vi "TCP IP Command Tester.vi"() -> ()   [LabVIEW 2015]
uses:
  Controls/Control_Fornax Set Monopolar Command - Coag Mode Enum.ctl
  Controls/Control_Fornax Set Monopolar Command - Serial Number String.ctl
  Controls/Control_Fornax Set Monopolar Command - Energy Channel ID Enum.ctl
  Controls/Control_Fornax Set Monopolar Command - Cut Mode Enum.ctl
  Controls/Control_Fornax Set Monopolar Command - Cut Power Command Enum.ctl
  Controls/Control_Fornax Set Monopolar Command - Coag Power Command Enum.ctl
  Controls/Control_Fornax Source ID.ctl
  Controls/Control_Fornax Switch ID.ctl
  Controls/Control_Fornax Energy Channel ID.ctl
  Controls/Control_Fornax Switch State.ctl
  Controls/Control_Fornax Energy Mode.ctl
  Controls/Control_Fornax Parameter Value.ctl
  Controls/Control_Fornax Parameter Type.ctl
  Controls/Control_Fornax Instrument Type.ctl
  Controls/Control_Fornax Mono1 Cut Increase Power.ctl
  Controls/Control_Fornax Mono1 Cut Decrease Power.ctl
  Controls/Control_Fornax Mono1 Coag Increase Power.ctl
  Controls/Control_Fornax Mono1 Coag Decrease Power.ctl
  Controls/Control_Fornax Mono1 Cut Enum.ctl
  Controls/Control_Fornax Mono1 Coag Enum.ctl
  Controls/Control_Fornax Mono1 Cut Activate Port Bool.ctl
  Controls/Control_Fornax Mono1 Coag Activate Port Bool.ctl
  Controls/Control_Fornax Mono2 Cut Activate Port Bool.ctl
  Controls/Control_Fornax Mono2 Coag Activate Port Bool.ctl
  Controls/Control_Fornax Mono2 Cut Decrease Power.ctl
  Controls/Control_Fornax Mono2 Cut Increase Power.ctl
  Controls/Control_Fornax Mono2 Cut Enum.ctl
  Controls/Control_Fornax Mono2 Coag Decrease Power.ctl
  Controls/Control_Fornax Mono2 Coag Increase Power.ctl
  Controls/Control_Fornax Mono2 Coag Enum.ctl
  Controls/Control_Fornax Bipolar Increase Power.ctl
  Controls/Control_Fornax Bipolar Decrease Power.ctl
  Controls/Control_Fornax Bipolar Enum.ctl
  Controls/Control_Fornax Bipolar Activate Port Bool.ctl
  Controls/Control_Fornax Ligasure Activate Port Bool.ctl
  Controls/QMH Fundamentals - Message Cluster.ctl
  Controls/Control_Fornax Generator.ctl
panel:
  in  "Stop":bool
  in  "Tab Control":T1(tab)
  in  "error in (no error)":errorcluster
  out "output cluster":T2
  out "Array":T3(array[cluster])
  in  "Fornax Executable Path":path=path "C:/Program Files (x86)/Medtronic/Fornax/x86/Fornax.exe"
  in  "Action 1":bool
  in  "ExternalCommCommand":T4(ring)=enum."EXTERNAL_COMM_COMMAND_PAIR_INTEGRATION_TESTOR"
  out "Display Message":string="Wait while TCP Connection established"
  in  "Set Monopolar Command":bool
  in  "CoagMode":T5
  in  "Serial Number":T6="T5G00443DX"
  in  "EnergyChannelID":T7
  in  "CutMode":T8
  in  "CutPowerCommand":T9
  in  "CoagPowerCommand":T10
  out "Display Message page 2":string="Wait while TCP Connection established"
  in  "String Command":string
  in  "Send String Command":bool
  out "String":string
  in  "Numeric (0-8)":i32
  in  "Send String Array Command":bool
  out "status":bool
  out "status 2":bool
  in  "Slider Status Command":bool
  in  "Switch Status Command":bool
  in  "System Config":bool
  in  "External Command":bool
  in  "External Command":T4(ring)
  in  "System Config":T11(ring)
  in  "Source ID":T12
  in  "Switch ID":T13
  in  "Switch State":T14
  in  "Energy Channel ID":T15
  in  "Energy Channel ID 2":T15
  in  "Slider Position":i32
  in  "Energy Parameter Command":bool
  in  "On/Off":bool
  in  "Mode":enum16{"Cut", "Coag", "Bipolar", "Ligasure"}(ring)
  in  "Port":enum16{"Mono1", "Mono2", "Bipolar", "Ligasure"}(ring)
  in  "Energy Mode":T16
  in  "Instrument Type":T17
  in  "Parameter Type":T18
  in  "Parameter Value":T19
  in  "Energy Channel ID 3":T15
  in  "Ligasure Activate":T20
  in  "Bipolar Activate":T21
  in  "Bipolar Enum":T22
  in  "Bipolar minus":T23
  in  "Bipolar plus":T24
  in  "Mono2 Coag Enum":T25=enum."Spray"
  in  "Mono2 Coag plus":T26
  in  "Mono2 Coag minus":T27
  in  "Mono2 Cut Enum":T28
  in  "Mono2 Cut plus":T29
  in  "Mono2 Cut minus":T30
  in  "Mono2 Coag Activate":T31
  in  "Mono2 Cut Activate":T32
  in  "Mono1 Coag Activate":T33
  in  "Mono1 Cut Activate":T34
  in  "Mono1 Coag Enum":T35=enum."Spray"
  in  "Mono1 Cut Enum":T36
  in  "Mono1 Coag minus":T37
  in  "Mono1 Coag plus":T38
  in  "Mono1 Cut minus":T39
  in  "Mono1 Cut plus":T40
  # "Mono1"
  # "Mono2"
  # "Bipolar"
  # "Ligasure"
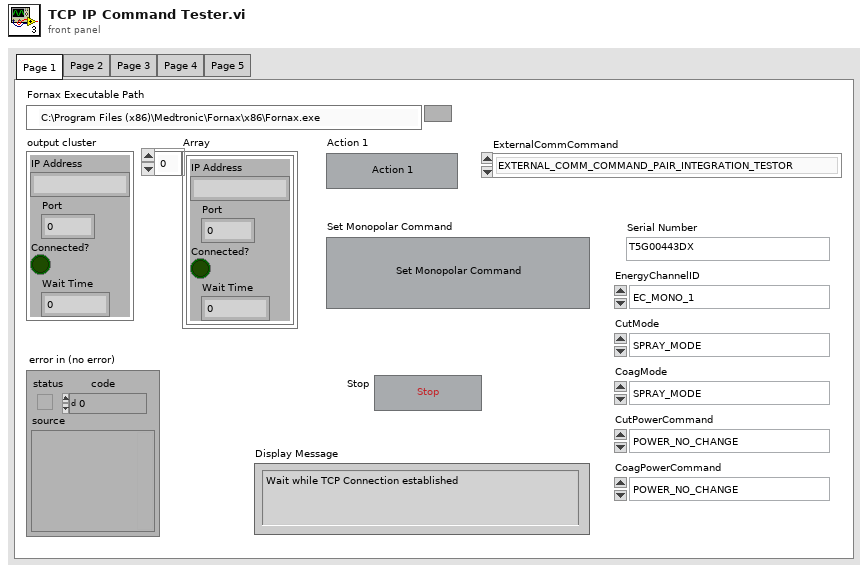
[diagram p1: front panel]
types:
  T1 = enum32{"Page 1", "Page 2", "Page 3", "Page 4", "Page 5"}
  T2 = cluster{"IP Address":string, "Port":u16, "Connected?":bool, "Wait Time":dbl}
  T3 = cluster{"IP Address":string, "Port":u16, "Connected?":bool, "Wait Time":dbl}[]
  T4 = enum16{"EXTERNAL_COMM_COMMAND_INVALID", "EXTERNAL_COMM_COMMAND_PAIR_VLEX", "EXTERNAL_COMM_COMMAND_PAIR_FORNAX", "EXTERNAL_COMM_COMMAND_PAIR_INTEGRATION_TESTOR", "EXTERNAL_COMM_COMMAND_ENABLE_DFA", "EXTERNAL_COMM_COMMAND_ENABLE_DFT", "EXTERNAL_COMM_COMMAND_ENABLE_VIPER", "EXTERNAL_COMM_COMMAND_AUTO_ETHERNET_ON", "EXTERNAL_COMM_COMMAND_AUTO_ETHERNET_OFF", "EXTERNAL_COMM_COMMAND_STREAM_RFDATA_ON", "EXTERNAL_COMM_COMMAND_STREAM_RFDATA_OFF", "EXTERNAL_COMM_COMMAND_STREAM_ISOFIRM_ON", "EXTERNAL_COMM_COMMAND_STREAM_ISOFIRM_OFF", "EXTERNAL_COMM_COMMAND_STREAM_RFID_ON", "EXTERNAL_COMM_COMMAND_STREAM_RFID_OFF", "EXTERNAL_COMM_COMMAND_AUTO_ETHERNET_ONCE"}
  T5 = typedef "Control_Fornax Set Monopolar Command - Coag Mode Enum.ctl" = enum16{"SPRAY_MODE", "CUT_MODE", "BLEND_MODE", "FULGERATE_MODE", "BEPOLAR_MODE", "VESSEL_SEALING_MODE", "VALLEYLAB_MODE", "BIPOLAR_RESECTION_CUT_MODE", "BIPOLAR_RESECTION_COAG_MODE", "AUTOBIPOLAR_MODE", "VIPER_HLA", "SOFT_COAG_MODE", "NUM_ENERGY_MODES"}
  T6 = typedef "Control_Fornax Set Monopolar Command - Serial Number String.ctl" = string
  T7 = typedef "Control_Fornax Set Monopolar Command - Energy Channel ID Enum.ctl" = enum16{"EC_MONO_1", "EC_BIPOLAR", "EC_MONO_2", "EC_ADVANCED", "NUM_ENERGY_CHANNELS", "EC_NOT_USED"}
  T8 = typedef "Control_Fornax Set Monopolar Command - Cut Mode Enum.ctl" = enum16{"SPRAY_MODE", "CUT_MODE", "BLEND_MODE", "FULGERATE_MODE", "BIPOLAR_MODE", "VESSEL_SEALING_MODE", "VALLEYLAB_MODE", "BIPOLAR_RESECTION_CUT_MODE", "BIPOLAR_RESECTION_COAG_MODE", "AUTOBIPOLAR_MODE", "VIPER_HLA", "SOFT_COAG_MODE", "NUM_ENERGY_MODES"}
  T9 = typedef "Control_Fornax Set Monopolar Command - Cut Power Command Enum.ctl" = enum16{"POWER_NO_CHANGE", "POWER_INCREASE", "POWER_DECREASE", "POWER_INCREASE_REPEAT", "POWER_DECREASE_REPEAT"}
  T10 = typedef "Control_Fornax Set Monopolar Command - Coag Power Command Enum.ctl" = enum16{"POWER_NO_CHANGE", "POWER_INCREASE", "POWER_DECREASE", "POWER_INCREASE_REPEAT", "POWER_DECREASE_REPEAT"}
  T11 = enum16{"SYSTEM_CONFIG_CMD_NONE", "SYSTEM_CONFIG_CMD_READ_CONFIG", "SYSTEM_CONFIG_CMD_WRITE_CONFIG", "SYSTEM_CONFIG_CMD_SW_UPDATE_ENTER", "SYSTEM_CONFIG_CMD_SW_UPDATE_START", "SYSTEM_CONFIG_CMD_SW_UPDATE_EXIT", "SYSTEM_CONFIG_CMD_UPDATE_ONE_BOARD_CHASSIS_INFO", "SYSTEM_CONFIG_CMD_UPDATE_ALL_BOARDS_CHASSIS_INFO", "SYSTEM_CONFIG_CMD_READ_ONE_BOARD_INFO", "SYSTEM_CONFIG_CMD_READ_ALL_BOARDS_INFO", "SYSTEM_CONFIG_CMD_REGISTER_BOARD", "SYSTEM_CONFIG_CMD_APPROVE_CURRENT_CONFIG", "SYSTEM_CONFIG_CMD_ROTATE_EVENT_LOGS", "SYSTEM_CONFIG_CMD_SYSTEM_RESTART", "SYSTEM_CONFIG_CMD_ROTATE_USAGE_LOGS", "SYSTEM_CONFIG_CMD_ENTER_SERVICE", "SYSTEM_CONFIG_CMD_EXIT_SERVICE", "SYSTEM_CONFIG_CMD_SW_UPDATE_CONFIRM", "SYSTEM_CONFIG_CMD_ROTATE_ALL_LOGS"}
  T12 = typedef "Control_Fornax Source ID.ctl" = enum16{"SWITCH_SOURCE_UNKNOWN  ", "SWITCH_SOURCE_HANDSWITCH  ", "SWITCH_SOURCE_FOOTSWITCH  ", "SWITCH_SOURCE_AUTO_BIPOLAR  ", "SWITCH_SOURCE_CARDIOBLATE  ", "SWITCH_SOURCE_SCREEN  ", "NUM_SWITCH_SOURCES  "}
  T13 = typedef "Control_Fornax Switch ID.ctl" = enum16{"SWITCH_ID_NONE  ", "SWITCH_ID_CUT  ", "SWITCH_ID_VMODE  ", "SWITCH_ID_COAG  ", "SWITCH_ID_LIGASURE  ", "SWITCH_ID_BIPOLAR  ", "SWITCH_ID_STAPLER_CLOSE  ", "SWITCH_ID_STAPLER_OPEN  ", "SWITCH_ID_CARDIOBLATE_BIPOLAR  ", "SWITCH_ID_CARDIOBLATE_BIPOLAR_TOUCHSCREEN  ", "SWITCH_ID_CARDIOBLATE_MONOPOLAR  ", "SWITCH_ID_CARDIOBLATE_MONOPOLAR_TOUCHSCREEN  ", "SWITCH_ID_ULTRASONIC_BTN1  ", "SWITCH_ID_ULTRASONIC_BTN2  ", "SWITCH_ID_MAX  "}
  T14 = typedef "Control_Fornax Switch State.ctl" = enum16{"SWITCH_STATE_NULL  ", "SWITCH_STATE_PRESSED  ", "SWITCH_STATE_RELEASED  ", "NUM_SWITCH_STATES  "}
  T15 = typedef "Control_Fornax Energy Channel ID.ctl" = enum16{"EC_MONO_1  ", "EC_BIPOLAR  ", "EC_MONO_2  ", "EC_ADVANCED  ", "EC_ADVANCED_ECUT  ", "EC_ADVANCED_DCUT  ", "EC_SHARED_COAG  ", "EC_INTERNAL_BIP_CAL  "}
  T16 = typedef "Control_Fornax Energy Mode.ctl" = enum16{"SPRAY_MODE", "CUT_MODE", "BLEND_MODE", "FULGERATE_MODE", "BIPOLAR_MODE", "VESSEL_SEALING_MODE", "VALLEYLAB_MODE", "BIPOLAR_RESECTION_CUT_MODE", "BIPOLAR_RESECTION_COAG_MODE", "AUTOBIPOLAR_MODE", "VIPER_HLA", "SOFT_COAG_MODE", "ECUT_MODE", "SHARED_SPRAY_MODE", "SHARED_FULGERATE_MODE", "CARDIO_MONO_MODE", "CARDIO_BIPOLAR_MODE", "BIPOLAR_LOW_MODE", "BIPOLAR_MACRO_MODE", "BIPOLAR_STANDARD_MODE", "BIPOLAR_MEDIUM_MODE", "VL_ENDOSCOPY_MODE", "NUM_ENERGY_MODES"}
  T17 = typedef "Control_Fornax Instrument Type.ctl" = enum16{"INSTRUMENT_TYPE_UNKNOWN", "INSTRUMENT_TYPE_MONOPOLAR", "INSTRUMENT_TYPE_BIPOLAR", "INSTRUMENT_TYPE_TRIVERSE", "INSTRUMENT_TYPE_LIGASURE", "INSTRUMENT_TYPE_ADVANCE_II", "INSTRUMENT_TYPE_BIPOLAR_RESECTION", "INSTRUMENT_TYPE_HOOK", "INSTRUMENT_TYPE_BIZACT", "INSTRUMENT_TYPE_CARDIOBLATE_BIP", "INSTRUMENT_TYPE_CARDIOBLATE_BIP_GEMINI_S", "INSTRUMENT_TYPE_CARDIOBLATE_MONO", "INSTRUMENT_TYPE_ULTRASONIC", "INSTRUMENT_TYPE_MONOPOLAR_GI ", "INSTRUMENT_TYPE_GOLDILOCKS "}
  T18 = typedef "Control_Fornax Parameter Type.ctl" = enum16{"POWER_PARAMETER", "CUT_MODALITY_POWER_PARAMETER", "COAG_MODALITY_POWER_PARAMETER", "VL_MODALITY_POWER_PARAMETER", "BY_MODE_POWER_PARAMETER", "VL_ENDO_CUT_MODALITY_POWER_PARAMETER", "VL_ENDO_COAG_MODALITY_POWER_PARAMETER", "VL_ENDO_COAG_ON_CUT_MODALITY_POWER_PARAMETER", "MODE_PARAMETER   (for changing Bipolar mode)", "CUT_MODALITY_MODE_PARAMETER  (for changing monopolar cut mode)", "COAG_MODALITY_MODE_PARAMETER (for changing monopolar coag mode)", "VL_ENDO_COAG_MODALITY_MODE_PARAMETER", "VL_ENDO_CUT_INTERVAL_PARAMETER", "VL_ENDO_CUT_DURATION_PARAMETER", "POWER_BAR_PARAMETER", "MAX_ACTIVATION_MSEC_TIME_PARAMETER", "AUTOBIPOLAR_DELAY_MSEC_TIME", "VL_ENDO_COAG_QUICK_ACCESS_PARAMETER"}
  T19 = typedef "Control_Fornax Parameter Value.ctl" = i32
  T20 = typedef "Control_Fornax Ligasure Activate Port Bool.ctl" = bool
  T21 = typedef "Control_Fornax Bipolar Activate Port Bool.ctl" = bool
  T22 = typedef "Control_Fornax Bipolar Enum.ctl" = enum16{"Standard", "Macro", "Precision"}
  T23 = typedef "Control_Fornax Bipolar Decrease Power.ctl" = bool
  T24 = typedef "Control_Fornax Bipolar Increase Power.ctl" = bool
  T25 = typedef "Control_Fornax Mono2 Coag Enum.ctl" = enum16{"Fulgerate", "Spray"}
  T26 = typedef "Control_Fornax Mono2 Coag Increase Power.ctl" = bool
  T27 = typedef "Control_Fornax Mono2 Coag Decrease Power.ctl" = bool
  T28 = typedef "Control_Fornax Mono2 Cut Enum.ctl" = enum16{"Pure", "Blend"}
  T29 = typedef "Control_Fornax Mono2 Cut Increase Power.ctl" = bool
  T30 = typedef "Control_Fornax Mono2 Cut Decrease Power.ctl" = bool
  T31 = typedef "Control_Fornax Mono2 Coag Activate Port Bool.ctl" = bool
  T32 = typedef "Control_Fornax Mono2 Cut Activate Port Bool.ctl" = bool
  T33 = typedef "Control_Fornax Mono1 Coag Activate Port Bool.ctl" = bool
  T34 = typedef "Control_Fornax Mono1 Cut Activate Port Bool.ctl" = bool
  T35 = typedef "Control_Fornax Mono1 Coag Enum.ctl" = enum16{"Fulgerate", "Spray"}
  T36 = typedef "Control_Fornax Mono1 Cut Enum.ctl" = enum16{"Pure", "Blend"}
  T37 = typedef "Control_Fornax Mono1 Coag Decrease Power.ctl" = bool
  T38 = typedef "Control_Fornax Mono1 Coag Increase Power.ctl" = bool
  T39 = typedef "Control_Fornax Mono1 Cut Decrease Power.ctl" = bool
  T40 = typedef "Control_Fornax Mono1 Cut Increase Power.ctl" = bool
  T41 = typedef "QMH Fundamentals - Message Cluster.ctl" = cluster{"Message":string, "Message Data":variant}
  T42 = cluster{"Port":enum16{"Mono1", "Mono2", "Bipolar", "Ligasure"}, "Mode":enum16{"Cut", "Coag", "Bipolar", "Ligasure"}, "On/Off":bool}
  T43 = typedef "Control_Fornax Generator.ctl" = string
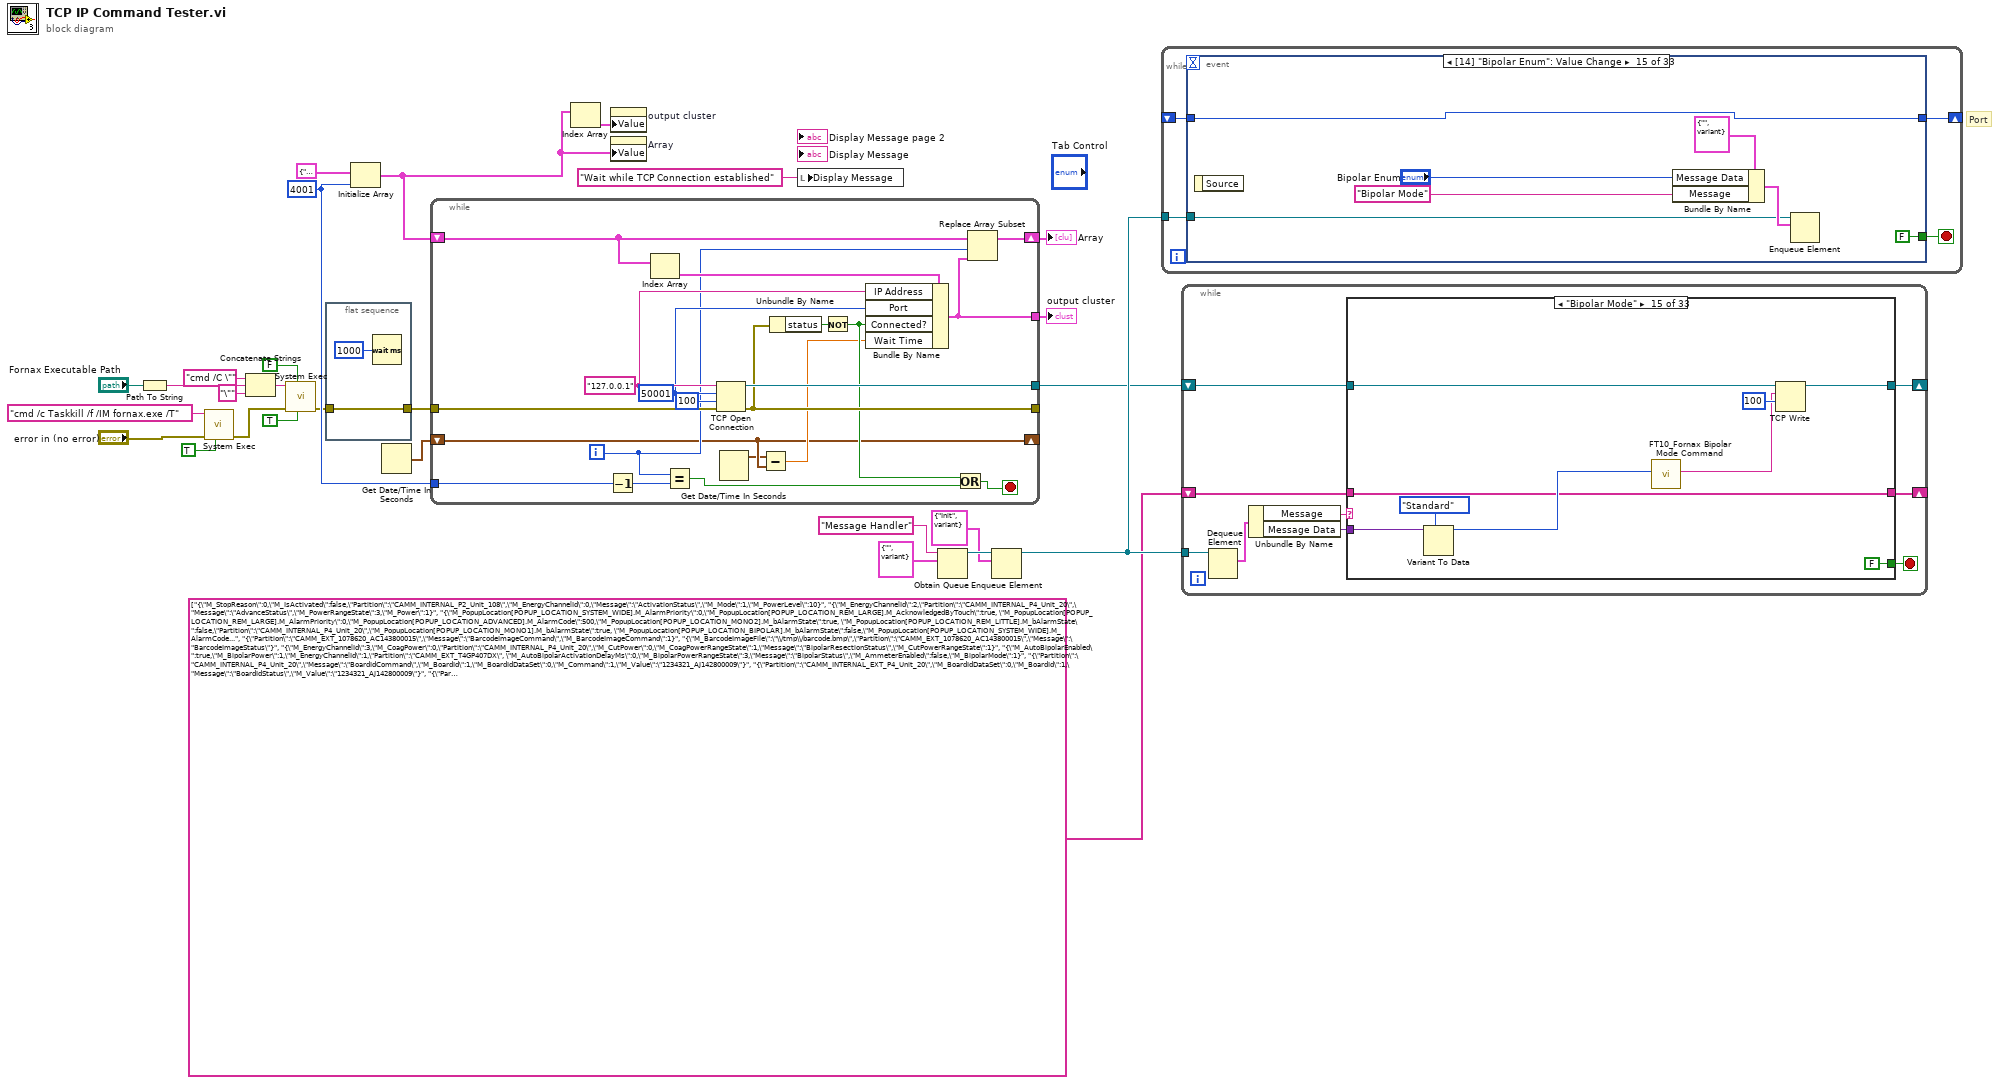
[diagram p0: block diagram]
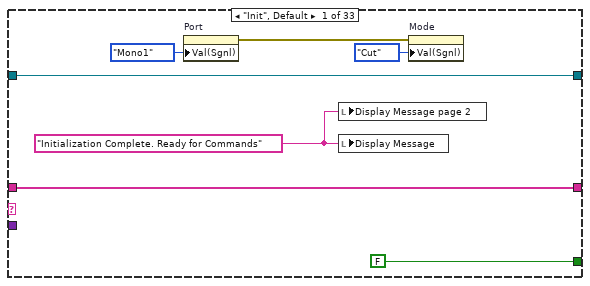
[diagram p2: hidden frame]
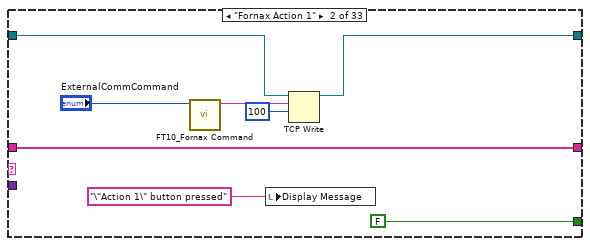
[diagram p3: hidden frame]
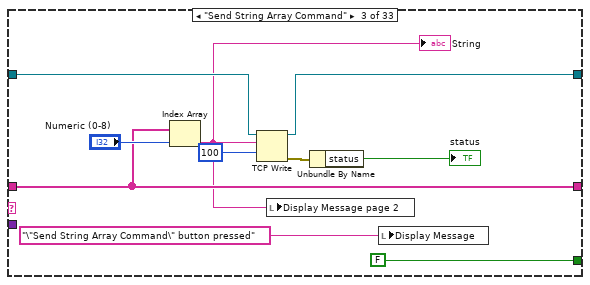
[diagram p4: hidden frame]
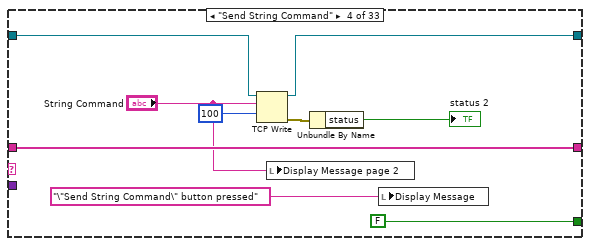
[diagram p5: hidden frame]
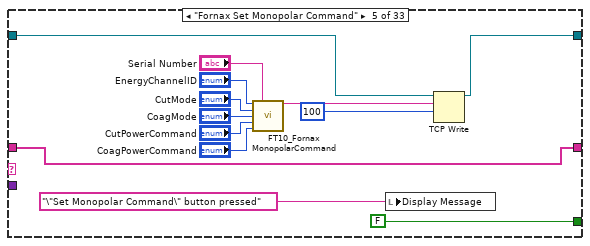
[diagram p6: hidden frame]
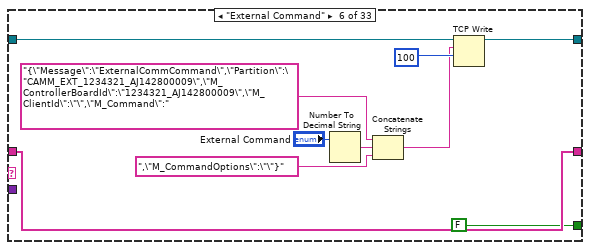
[diagram p7: hidden frame]
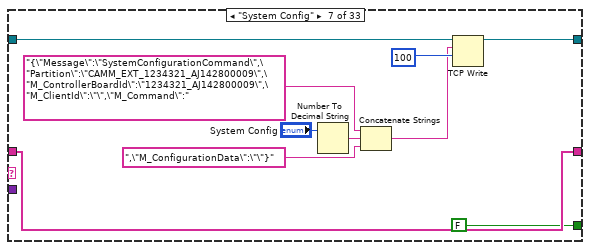
[diagram p8: hidden frame]
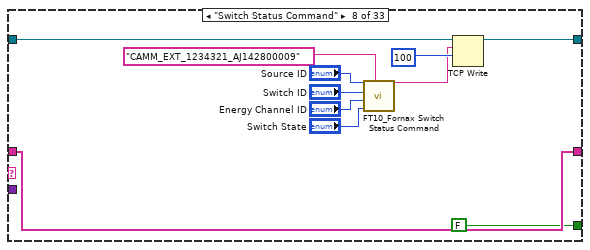
[diagram p9: hidden frame]
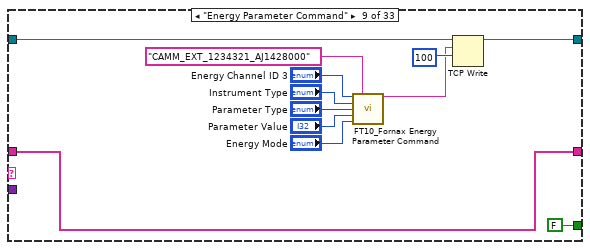
[diagram p10: hidden frame]
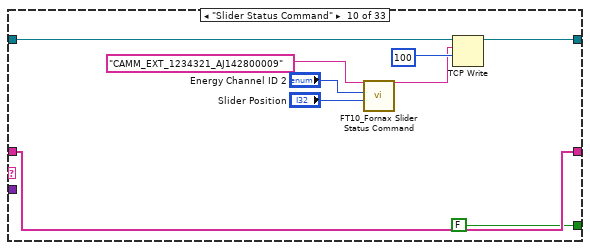
[diagram p11: hidden frame]
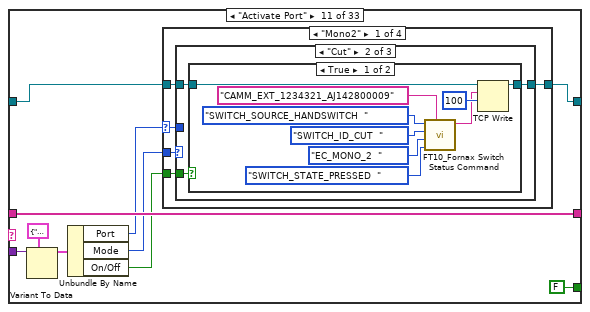
[diagram p12: hidden frame]
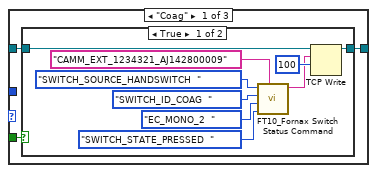
[diagram p13: hidden frame]
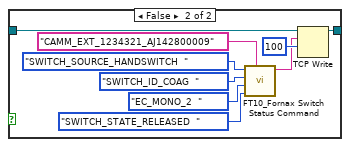
[diagram p14: hidden frame]
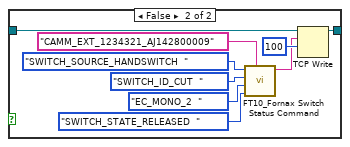
[diagram p15: hidden frame]
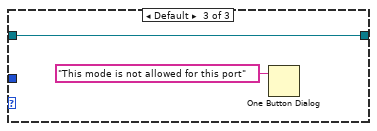
[diagram p16: hidden frame]
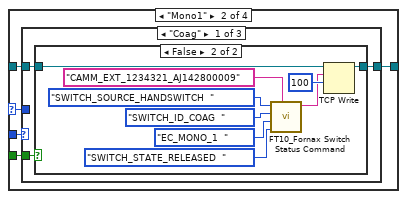
[diagram p17: hidden frame]
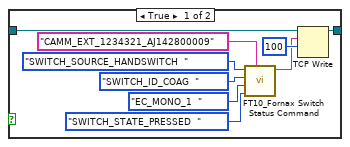
[diagram p18: hidden frame]
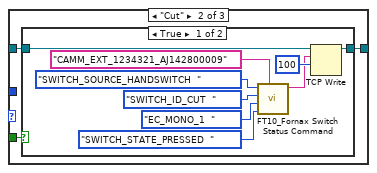
[diagram p19: hidden frame]
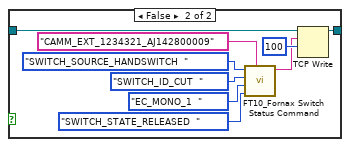
[diagram p20: hidden frame]
diagram:
  w26 = 4001 ("dimension size")
  # "Port"
  n1 = Path To String(path="Fornax Executable Path") -> (string=w15:string)
  n2 = call <vilib>:"System Exec.vi"("run minimized? (F)"=TRUE, "error in (no error)"="error in (no error)", "command line"="cmd /c Taskkill /f /IM fornax.exe /T") -> ("error out"=w21:errorcluster)  [unwired: 5 in, 3 out]
  n3 = Concatenate Strings("cmd /C \"" ("string"), w15, "\"" ("string")) -> (w17:string)
  n4 = call <vilib>:"System Exec.vi"("run minimized? (F)"=TRUE, "wait until completion? (T)"=FALSE, "error in (no error)"=w21, "command line"=w17) -> ("error out"=w1:errorcluster)  [unwired: 4 in, 3 out]
  n5 = flat-sequence {
    tunnel: [w30] -> w2
    tunnel: w1 -> [w30]
    frame #0 {
      n6 = Wait (ms)(milliseconds to wait=u32 1000) -> ()  [unwired: 1 out]
    }
  }
  n7 = Initialize Array(T2 {"IP Address"="", "Port"=0, "Connected?"=FALSE, "Wait Time"=0.0} ("Cluster"), w26) -> (w4:T3)
  n8 = Get Date/Time In Seconds() -> (seconds since 1Jan1904=w23:timestamp)
  n9 = while {
    tunnel: [w49] -> w7
    shift-right: [w48] -> w24
    shift-left: w4 -> [w47]
    tunnel: w26 -> [w38]
    tunnel: [w35] -> w25
    shift-right: [w32] -> _
    shift-left: w23 -> [w32]
    tunnel: w2 -> [w50]
    tunnel: [w43] -> _
    i -> [w34]
    stop <- w40 stop-if-true
    w44 = u16 50001 ("remote port or service name")
    w45 = "127.0.0.1" ("address")
    n10 = Decrement(x=w38) -> (x-1=w37:i32)
    n11 = Index Array(array=w47) -> (element=w46:T2)  [unwired: 1 in]
    n12 = Equal?(x=w34, y=w37) -> (x = y?=w36:bool)
    n13 = TCP Open Connection(address=w45, remote port or service name=w44, timeout ms (60000)=100, error in (no error)=w50) -> (connection ID=w49:refnum<k5>, error out=w43:errorcluster)  [unwired: 1 in]
    n14 = Get Date/Time In Seconds() -> (seconds since 1Jan1904=w31:timestamp)
    n15 = Subtract(x=w31, y=w32) -> (x-y=w33:dbl)
    n16 = Unbundle By Name(w43) -> ("status"=w42:bool)
    n17 = Not(x=w42) -> (.not. x?=w39:bool)
    n18 = Bundle By Name(cluster=w46, "IP Address"=w45, "Port"=w44, "Connected?"=w39, "Wait Time"=w33) -> (w35:T2)
    n19 = Or(x=w39, y=w36) -> (x .or. y?=w40:bool)
    n20 = Replace Array Subset(array=w47, new element=w35, index=w34) -> (w48:T3)
  }
  "output cluster" <- w25
  "Array" <- w24
  n21 = Index Array(array=w4) -> (element=w5:T2)  [unwired: 1 in]
  n22 = property on="output cluster" class="Clust (strict)"("Value"=w5) -> ()  [unwired: 2 in, 2 out]
  n23 = property on="Array" class="Arr (strict)"("Value"=w4) -> ()  [unwired: 2 in, 2 out]
  n24 = local write "Display Message"("Wait while TCP Connection established" ("Display Message")) -> ()
  n25 = Obtain Queue(name (unnamed)="Message Handler", element data type=T41 {"Message"="", "Message Data"=variant} ("Message Cluster")) -> (queue out=w11:refnum<queue>)  [unwired: 3 in, 2 out]
  n26 = Enqueue Element(queue=w11, element=T41 {"Message"="Init", "Message Data"=variant}) -> (queue out=w8:refnum<queue>)  [unwired: 2 in, 2 out]
  n27 = while {
    tunnel: w8 -> [w54]
    shift-right: [w52] -> _
    shift-left: _ -> [w51]
    stop <- w53 stop-if-true
    n28 = event shown="[14] \"Bipolar Enum\": Value Change" {
      selector: _ -> [_ _ _ _ _ _ _ _ _ _ _ _ _ _ _ _ _ _ _ _ _ _ _ _ _ _ _ _ _ _ _ _ _]
      dyn-events: _ -> [_ _ _ _ _ _ _ _ _ _ _ _ _ _ _ _ _ _ _ _ _ _ _ _ _ _ _ _ _ _ _ _ _]
      timeout: _ -> [_ _ _ _ _ _ _ _ _ _ _ _ _ _ _ _ _ _ _ _ _ _ _ _ _ _ _ _ _ _ _ _ _]
      tunnel: w54 -> [w57 w61 w65 w69 w75 w81 w87 w93 w99 _ w115 w126 w135 w142 w149 w157 w166 w173 w180 w188 w197 w204 w211 w219 w228 w235 w242 w250 w259 w266 w273 w281 w289]
      tunnel: [FALSE FALSE FALSE FALSE FALSE FALSE FALSE FALSE FALSE FALSE FALSE FALSE FALSE FALSE FALSE FALSE FALSE FALSE FALSE FALSE FALSE FALSE FALSE FALSE FALSE FALSE FALSE FALSE FALSE FALSE FALSE FALSE TRUE] -> w53
      tunnel: [w55 w59 w63 w67 w71 w77 w83 w89 w95 w102 w113 w123 w133 w140 w146 w154 w164 w171 w178 w185 w195 w202 w209 w216 w226 w233 w240 w247 w257 w264 w271 w278 w287] -> w52
      tunnel: w51 -> [w55 w59 w63 w67 w71 w77 w83 w89 w95 _ w113 w123 w133 w140 w146 w154 w164 w171 w178 w185 w195 w202 w209 w216 w226 w233 w240 w247 w257 w264 w271 w278 w287]
      event "Action 1": Value Change {
        n29 = event-data() -> ()  [unwired: 1 in, 4 out]
        n30 = Enqueue Element(queue=w57, element=T41 {"Message"="Fornax Action 1", "Message Data"=variant}) -> ()  [unwired: 2 in, 3 out]
      }
      event "Set Monopolar Command": Value Change {
        n31 = event-data() -> ()  [unwired: 1 in, 2 out]
        n32 = Enqueue Element(queue=w61, element=T41 {"Message"="Fornax Set Monopolar Command", "Message Data"=variant}) -> ()  [unwired: 2 in, 3 out]
      }
      event "Send String Array Command": Value Change {
        n33 = event-data() -> ()  [unwired: 1 in, 3 out]
        n34 = Enqueue Element(queue=w65, element=T41 {"Message"="Send String Array Command", "Message Data"=variant}) -> ()  [unwired: 2 in, 3 out]
      }
      event "Send String Command": Value Change {
        n35 = event-data() -> ()  [unwired: 1 in, 2 out]
        n36 = Enqueue Element(queue=w69, element=T41 {"Message"="Send String Command", "Message Data"=variant}) -> ()  [unwired: 2 in, 3 out]
      }
      event "External Command": Value Change {
        n37 = event-data() -> ()  [unwired: 1 in, 4 out]
        n38 = Bundle By Name(cluster=T41 {"Message"="", "Message Data"=variant} ("element"), "Message"="External Command") -> (w73:T41)
        n39 = Enqueue Element(queue=w75, element=w73) -> ()  [unwired: 2 in, 3 out]
      }
      event "System Config": Value Change {
        n40 = event-data() -> ()  [unwired: 1 in, 3 out]
        n41 = Bundle By Name(cluster=T41 {"Message"="", "Message Data"=variant} ("element"), "Message"="System Config") -> (w79:T41)
        n42 = Enqueue Element(queue=w81, element=w79) -> ()  [unwired: 2 in, 3 out]
      }
      event "Switch Status Command": Value Change {
        n43 = event-data() -> ()  [unwired: 1 in, 3 out]
        n44 = Bundle By Name(cluster=T41 {"Message"="", "Message Data"=variant} ("element"), "Message"="Switch Status Command") -> (w85:T41)
        n45 = Enqueue Element(queue=w87, element=w85) -> ()  [unwired: 2 in, 3 out]
      }
      event "Slider Status Command": Value Change {
        n46 = event-data() -> ()  [unwired: 1 in, 2 out]
        n47 = Bundle By Name(cluster=T41 {"Message"="", "Message Data"=variant} ("element"), "Message"="Slider Status Command") -> (w91:T41)
        n48 = Enqueue Element(queue=w93, element=w91) -> ()  [unwired: 2 in, 3 out]
      }
      event "Energy Parameter Command": Value Change {
        n49 = event-data() -> ()  [unwired: 1 in, 1 out]
        n50 = Bundle By Name(cluster=T41 {"Message"="", "Message Data"=variant} ("element"), "Message"="Energy Parameter Command") -> (w97:T41)
        n51 = Enqueue Element(queue=w99, element=w97) -> ()  [unwired: 2 in, 3 out]
      }
      event "Port": Value Change {
        n52 = event-data() -> ()  [unwired: 1 in, 1 out]
        n53 = case shown="\"Ligasure\"" "Port" {
          selector: "Port" -> [w104 w106 w108 w110]
          tunnel: [w104 w106 w108 w110] -> w102
          frame "Mono1", Default {
            # "Modes:\n0 - Cut\n1 - Coag\n2 - Bipolar\n3 - Ligasure"
            n54 = property on="Mode" class="Enum (strict)"("Disabled Items []"=i32[] [2, 3]) -> ()  [unwired: 2 in, 2 out]
          }
          frame "Mono2" {
            # "Modes:\n0 - Cut\n1 - Coag\n2 - Bipolar\n3 - Ligasure"
            n55 = property on="Mode" class="Enum (strict)"("Disabled Items []"=i32[] [2, 3]) -> ()  [unwired: 2 in, 2 out]
          }
          frame "Bipolar" {
            # "Modes:\n0 - Cut\n1 - Coag\n2 - Bipolar\n3 - Ligasure"
            n56 = property on="Mode" class="Enum (strict)"("Disabled Items []"=i32[] [0, 1, 3]) -> ()  [unwired: 2 in, 2 out]
          }
          frame "Ligasure" {
            # "Modes:\n0 - Cut\n1 - Coag\n2 - Bipolar\n3 - Ligasure"
            n57 = property on="Mode" class="Enum (strict)"("Disabled Items []"=i32[] [0, 1, 2]) -> ()  [unwired: 2 in, 2 out]
          }
        }
      }
      event "On/Off": Value Change {
        n58 = event-data() -> ()  [unwired: 1 in, 1 out]
        n59 = Bundle By Name(cluster=T42 {"Port"=enum."Bipolar", "Mode"=enum."Bipolar", "On/Off"=FALSE}, "Port"=w113, "Mode"="Mode", "On/Off"="On/Off") -> (w114:T42)
        n60 = Bundle By Name(cluster=T41 {"Message"="", "Message Data"=variant} ("element"), "Message Data"=w114, "Message"="Activate Port") -> (w117:T41)
        n61 = Enqueue Element(queue=w115, element=w117) -> ()  [unwired: 2 in, 3 out]
      }
      event Value Change {
        n62 = event-data() -> ()  [unwired: 1 in, 1 out]
        n63 = case shown="True" "Bipolar Activate" {
          tunnel: ["Deactivate" ("Message") "Activate" ("Message")] -> w125
          frame True {
          }
          frame False {
          }
        }
        n64 = property on="Bipolar Activate" class="Bool (strict)"("BoolText.Text"=w125) -> ()  [unwired: 2 in, 2 out]
        n65 = Bundle By Name(cluster=T41 {"Message"="", "Message Data"=variant} ("element"), "Message Data"="Bipolar Activate", "Message"="Bipolar Activate Port") -> (w128:T41)
        n66 = Enqueue Element(queue=w126, element=w128) -> ()  [unwired: 2 in, 3 out]
      }
      event Value Change {
        n67 = event-data() -> ()  [unwired: 1 in, 1 out]
        n68 = Bundle By Name(cluster=T41 {"Message"="", "Message Data"=variant} ("element"), "Message Data"="Bipolar minus", "Message"="Bipolar Decrease Power") -> (w137:T41)
        n69 = Enqueue Element(queue=w135, element=w137) -> ()  [unwired: 2 in, 3 out]
      }
      event Value Change {
        n70 = event-data() -> ()  [unwired: 1 in, 1 out]
        n71 = Bundle By Name(cluster=T41 {"Message"="", "Message Data"=variant} ("element"), "Message Data"="Bipolar plus", "Message"="Bipolar Increase Power") -> (w144:T41)
        n72 = Enqueue Element(queue=w142, element=w144) -> ()  [unwired: 2 in, 3 out]
      }
      event Value Change {
        n73 = event-data() -> ()  [unwired: 1 in, 1 out]
        n74 = Bundle By Name(cluster=T41 {"Message"="", "Message Data"=variant} ("element"), "Message Data"="Bipolar Enum", "Message"="Bipolar Mode") -> (w151:T41)
        n75 = Enqueue Element(queue=w149, element=w151) -> ()  [unwired: 2 in, 3 out]
      }
      event Value Change {
        n76 = event-data() -> ()  [unwired: 1 in, 4 out]
        n77 = case shown="True" "Mono1 Cut Activate" {
          tunnel: ["Deactivate" ("Message") "Activate" ("Message")] -> w156
          frame True {
          }
          frame False {
          }
        }
        n78 = property on="Mono1 Cut Activate" class="Bool (strict)"("BoolText.Text"=w156) -> ()  [unwired: 2 in, 2 out]
        n79 = Bundle By Name(cluster=T41 {"Message"="", "Message Data"=variant} ("element"), "Message Data"="Mono1 Cut Activate", "Message"="Mono1 Cut Activate Port") -> (w159:T41)
        n80 = Enqueue Element(queue=w157, element=w159) -> ()  [unwired: 2 in, 3 out]
      }
      event Value Change {
        n81 = event-data() -> ()  [unwired: 1 in, 4 out]
        n82 = Bundle By Name(cluster=T41 {"Message"="", "Message Data"=variant} ("element"), "Message Data"="Mono1 Cut minus", "Message"="Mono1 Cut Decrease Power") -> (w168:T41)
        n83 = Enqueue Element(queue=w166, element=w168) -> ()  [unwired: 2 in, 3 out]
      }
      event Value Change {
        n84 = event-data() -> ()  [unwired: 1 in, 4 out]
        n85 = Bundle By Name(cluster=T41 {"Message"="", "Message Data"=variant} ("element"), "Message Data"="Mono1 Cut plus", "Message"="Mono1 Cut Increase Power") -> (w175:T41)
        n86 = Enqueue Element(queue=w173, element=w175) -> ()  [unwired: 2 in, 3 out]
      }
      event Value Change {
        n87 = event-data() -> ()  [unwired: 1 in, 4 out]
        n88 = Bundle By Name(cluster=T41 {"Message"="", "Message Data"=variant} ("element"), "Message Data"="Mono1 Cut Enum", "Message"="Mono1 Cut Mode") -> (w182:T41)
        n89 = Enqueue Element(queue=w180, element=w182) -> ()  [unwired: 2 in, 3 out]
      }
      event Value Change {
        n90 = event-data() -> ()  [unwired: 1 in, 4 out]
        n91 = case shown="True" "Mono1 Coag Activate" {
          tunnel: ["Deactivate" ("Message") "Activate" ("Message")] -> w186
          frame True {
          }
          frame False {
          }
        }
        n92 = property on="Mono1 Coag Activate" class="Bool (strict)"("BoolText.Text"=w186) -> ()  [unwired: 2 in, 2 out]
        n93 = Bundle By Name(cluster=T41 {"Message"="", "Message Data"=variant} ("element"), "Message Data"="Mono1 Coag Activate", "Message"="Mono1 Coag Activate Port") -> (w190:T41)
        n94 = Enqueue Element(queue=w188, element=w190) -> ()  [unwired: 2 in, 3 out]
      }
      event Value Change {
        n95 = event-data() -> ()  [unwired: 1 in, 4 out]
        n96 = Bundle By Name(cluster=T41 {"Message"="", "Message Data"=variant} ("element"), "Message Data"="Mono1 Coag minus", "Message"="Mono1 Coag Decrease Power") -> (w199:T41)
        n97 = Enqueue Element(queue=w197, element=w199) -> ()  [unwired: 2 in, 3 out]
      }
      event Value Change {
        n98 = event-data() -> ()  [unwired: 1 in, 4 out]
        n99 = Bundle By Name(cluster=T41 {"Message"="", "Message Data"=variant} ("element"), "Message Data"="Mono1 Coag plus", "Message"="Mono1 Coag Increase Power") -> (w206:T41)
        n100 = Enqueue Element(queue=w204, element=w206) -> ()  [unwired: 2 in, 3 out]
      }
      event Value Change {
        n101 = event-data() -> ()  [unwired: 1 in, 4 out]
        n102 = Bundle By Name(cluster=T41 {"Message"="", "Message Data"=variant} ("element"), "Message Data"="Mono1 Coag Enum", "Message"="Mono1 Coag Mode") -> (w213:T41)
        n103 = Enqueue Element(queue=w211, element=w213) -> ()  [unwired: 2 in, 3 out]
      }
      event Value Change {
        n104 = event-data() -> ()  [unwired: 1 in, 4 out]
        n105 = case shown="True" "Mono2 Cut Activate" {
          tunnel: ["Deactivate" ("Message") "Activate" ("Message")] -> w218
          frame True {
          }
          frame False {
          }
        }
        n106 = property on="Mono2 Cut Activate" class="Bool (strict)"("BoolText.Text"=w218) -> ()  [unwired: 2 in, 2 out]
        n107 = Bundle By Name(cluster=T41 {"Message"="", "Message Data"=variant} ("element"), "Message Data"="Mono2 Cut Activate", "Message"="Mono2 Cut Activate Port") -> (w221:T41)
        n108 = Enqueue Element(queue=w219, element=w221) -> ()  [unwired: 2 in, 3 out]
      }
      event Value Change {
        n109 = event-data() -> ()  [unwired: 1 in, 4 out]
        n110 = Bundle By Name(cluster=T41 {"Message"="", "Message Data"=variant} ("element"), "Message Data"="Mono2 Cut minus", "Message"="Mono2 Cut Decrease Power") -> (w230:T41)
        n111 = Enqueue Element(queue=w228, element=w230) -> ()  [unwired: 2 in, 3 out]
      }
      event Value Change {
        n112 = event-data() -> ()  [unwired: 1 in, 4 out]
        n113 = Bundle By Name(cluster=T41 {"Message"="", "Message Data"=variant} ("element"), "Message Data"="Mono2 Cut plus", "Message"="Mono2 Cut Increase Power") -> (w237:T41)
        n114 = Enqueue Element(queue=w235, element=w237) -> ()  [unwired: 2 in, 3 out]
      }
      event Value Change {
        n115 = event-data() -> ()  [unwired: 1 in, 4 out]
        n116 = Bundle By Name(cluster=T41 {"Message"="", "Message Data"=variant} ("element"), "Message Data"="Mono2 Cut Enum", "Message"="Mono2 Cut Mode") -> (w244:T41)
        n117 = Enqueue Element(queue=w242, element=w244) -> ()  [unwired: 2 in, 3 out]
      }
      event Value Change {
        n118 = event-data() -> ()  [unwired: 1 in, 4 out]
        n119 = case shown="True" "Mono2 Coag Activate" {
          tunnel: ["Deactivate" ("Message") "Activate" ("Message")] -> w249
          frame True {
          }
          frame False {
          }
        }
        n120 = property on="Mono2 Coag Activate" class="Bool (strict)"("BoolText.Text"=w249) -> ()  [unwired: 2 in, 2 out]
        n121 = Bundle By Name(cluster=T41 {"Message"="", "Message Data"=variant} ("element"), "Message Data"="Mono2 Coag Activate", "Message"="Mono2 Coag Activate Port") -> (w252:T41)
        n122 = Enqueue Element(queue=w250, element=w252) -> ()  [unwired: 2 in, 3 out]
      }
      event Value Change {
        n123 = event-data() -> ()  [unwired: 1 in, 4 out]
        n124 = Bundle By Name(cluster=T41 {"Message"="", "Message Data"=variant} ("element"), "Message Data"="Mono2 Coag minus", "Message"="Mono2 Coag Decrease Power") -> (w261:T41)
        n125 = Enqueue Element(queue=w259, element=w261) -> ()  [unwired: 2 in, 3 out]
      }
      event Value Change {
        n126 = event-data() -> ()  [unwired: 1 in, 4 out]
        n127 = Bundle By Name(cluster=T41 {"Message"="", "Message Data"=variant} ("element"), "Message Data"="Mono2 Coag plus", "Message"="Mono2 Coag Increase Power") -> (w268:T41)
        n128 = Enqueue Element(queue=w266, element=w268) -> ()  [unwired: 2 in, 3 out]
      }
      event Value Change {
        n129 = event-data() -> ()  [unwired: 1 in, 4 out]
        n130 = Bundle By Name(cluster=T41 {"Message"="", "Message Data"=variant} ("element"), "Message Data"="Mono2 Coag Enum", "Message"="Mono2 Coag Mode") -> (w275:T41)
        n131 = Enqueue Element(queue=w273, element=w275) -> ()  [unwired: 2 in, 3 out]
      }
      event Value Change {
        n132 = event-data() -> ()  [unwired: 1 in, 4 out]
        n133 = case shown="True" "Ligasure Activate" {
          tunnel: ["Deactivate" ("Message") "Activate" ("Message")] -> w279
          frame True {
          }
          frame False {
          }
        }
        n134 = property on="Ligasure Activate" class="Bool (strict)"("BoolText.Text"=w279) -> ()  [unwired: 2 in, 2 out]
        n135 = Bundle By Name(cluster=T41 {"Message"="", "Message Data"=variant} ("element"), "Message Data"="Ligasure Activate", "Message"="Ligasure Activate Port") -> (w283:T41)
        n136 = Enqueue Element(queue=w281, element=w283) -> ()  [unwired: 2 in, 3 out]
      }
      event "Stop": Value Change {
        n137 = event-data() -> ()  [unwired: 1 in, 5 out]
        n138 = Enqueue Element At Opposite End(queue=w289, element=T41 {"Message"="Exit", "Message Data"=variant}) -> ()  [unwired: 2 in, 3 out]
      }
    }
  }
  n139 = while {
    tunnel: w8 -> [w298]
    shift-right: [w295] -> _
    shift-left: w7 -> [w294]
    shift-right: [w292] -> _
    shift-left: string[] ["{\"M_StopReason\":0,\"M_IsActivated\":false,\"Partition\":\"CAMM_INTERNAL_P2_Unit_108\",\"M_EnergyChannelId\":0,\"Message\":\"ActivationStatus\",\"M_Mode\":1,\"M_PowerLevel\":10}", "{\"M_EnergyChannelId\":2,\"Partition\":\"CAMM_INTERNAL_P4_Unit_20\",\"Message\":\"AdvanceStatus\",\"M_PowerRangeState\":3,\"M_Power\":1}", "{\"M_PopupLocation[POPUP_LOCATION_SYSTEM_WIDE].M_AlarmPriority\":0,\"M_PopupLocation[POPUP_LOCATION_REM_LARGE].M_AcknowledgedByTouch\":true, \"M_PopupLocation[POPUP_LOCATION_REM_LARGE].M_AlarmPriority\":0,\"M_PopupLocation[POPUP_LOCATION_ADVANCED].M_AlarmCode\":500,\"M_PopupLocation[POPUP_LOCATION_MONO2].M_bAlarmState\":true, \"M_PopupLocation[POPUP_LOCATION_REM_LITTLE].M_bAlarmState\":false,\"Partition\":\"CAMM_INTERNAL_P4_Unit_20\",\"M_PopupLocation[POPUP_LOCATION_MONO1].M_bAlarmState\":true, \"M_PopupLocation[POPUP_LOCATION_BIPOLAR].M_bAlarmState\":false,\"M_PopupLocation[POPUP_LOCATION_SYSTEM_WIDE].M_AlarmCode\":500,\"M_PopupLocation[POPUP_LOCATION_DEMO_MODE].M_AlarmCode\":500, \"M_PopupLocation[POPUP_LOCATION_SYSTEM_WIDE].M_AcknowledgedByTouch\":true,\"M_PopupLocation[POPUP_LOCATION_ADVANCED].M_AcknowledgedByTouch\":true, \"M_PopupLocation[POPUP_LOCATION_REM_LARGE].M_bAlarmState\":false,\"M_PopupLocation[POPUP_LOCATION_REM_LITTLE].M_AcknowledgedByTouch\":false,\"M_PopupLocation[POPUP_LOCATION_BIPOLAR].M_AlarmCode\":500, \"M_PopupLocation[POPUP_LOCATION_MONO1].M_AcknowledgedByTouch\":true,\"M_PopupLocation[POPUP_LOCATION_MONO1].M_AlarmCode\":331,\"M_PopupLocation[POPUP_LOCATION_REM_LITTLE].M_AlarmPriority\":0, \"Message\":\"AlarmPopupStatus\",\"M_PopupLocation[POPUP_LOCATION_DEMO_MODE].M_AcknowledgedByTouch\":true,\"M_PopupLocation[POPUP_LOCATION_MONO2].M_AlarmCode\":331, \"M_PopupLocation[POPUP_LOCATION_ADVANCED].M_AlarmPriority\":0,\"M_PopupLocation[POPUP_LOCATION_REM_LITTLE].M_AlarmCode\":500,\"M_PopupLocation[POPUP_LOCATION_BIPOLAR].M_AcknowledgedByTouch\":true, \"M_PopupLocation[POPUP_LOCATION_MONO1].M_AlarmPriority\":3,\"M_PopupLocation[POPUP_LOCATION_REM_LARGE].M_AlarmCode\":500,\"M_PopupLocation[POPUP_LOCATION_DEMO_MODE].M_bAlarmState\":false, \"M_PopupLocation[POPUP_LOCATION_SYSTEM_WIDE].M_bAlarmState\":false,\"M_PopupLocation[POPUP_LOCATION_MONO2].M_AcknowledgedByTouch\":true, \"M_PopupLocation[POPUP_LOCATION_BIPOLAR].M_AlarmPriority\":0,\"M_PopupLocation[POPUP_LOCATION_ADVANCED].M_bAlarmState\":false, \"M_PopupLocation[POPUP_LOCATION_DEMO_MODE].M_AlarmPriority\":0,\"M_PopupLocation[POPUP_LOCATION_MONO2].M_AlarmPriority\":3}", "{\"Partition\":\"CAMM_EXT_1078620_AC143800015\",\"Message\":\"BarcodeImageCommand\",\"M_BarcodeImageCommand\":1}", "{\"M_BarcodeImageFile\":\"\\/tmp\\/barcode.bmp\",\"Partition\":\"CAMM_EXT_1078620_AC143800015\",\"Message\":\"BarcodeImageStatus\"}", "{\"M_EnergyChannelId\":3,\"M_CoagPower\":0,\"Partition\":\"CAMM_INTERNAL_P4_Unit_20\",\"M_CutPower\":0,\"M_CoagPowerRangeState\":1,\"Message\":\"BipolarResectionStatus\",\"M_CutPowerRangeState\":1}", "{\"M_AutoBipolarEnabled\":true,\"M_BipolarPower\":1,\"M_EnergyChannelId\":1,\"Partition\":\"CAMM_EXT_T4GP407DX\", \"M_AutoBipolarActivationDelayMs\":0,\"M_BipolarPowerRangeState\":3,\"Message\":\"BipolarStatus\",\"M_AmmeterEnabled\":false,\"M_BipolarMode\":1}", "{\"Partition\":\"CAMM_INTERNAL_P4_Unit_20\",\"Message\":\"BoardIdCommand\",\"M_BoardId\":1,\"M_BoardIdDataSet\":0,\"M_Command\":1,\"M_Value\":\"1234321_AJ142800009\"}", "{\"Partition\":\"CAMM_INTERNAL_EXT_P4_Unit_20\",\"M_BoardIdDataSet\":0,\"M_BoardId\":1,\"Message\":\"BoardIdStatus\",\"M_Value\":\"1234321_AJ142800009\"}", "{\"Partition\":\"CAMM_INTERNAL_EXT_P4_Unit_20\",\"Message\":\"CardioblateBipolarStatus\",\"M_EnergyChannelId\":3,\"M_MaximumAblationTimeMS\":5,\"M_MaximumPowerLevel\":5}", "{\"Partition\":\"CAMM_INTERNAL_EXT_P4_Unit_20\",\"Message\":\"CardioblateMonopolarStatus\",\"M_CardioblateMonopolarPower\":5, \"M_CardioblateMonopolarPowerRangeState\":3,\"M_MaximumActivationTimeMS\":10,\"M_MaximumActivationTimeMSRangeState\":3}", "{\"Partition\":\"CAMM_INTERNAL_EXT_P4_Unit_20\",\"Message\":\"CardioblateSelectStatus\",\"M_SelectedEnergyChannel\":3}", "{\"Partition\":\"CAMM_EXT_1078620_AC143800015\",\"Message\":\"DftAlarmCommand\",\"M_ModuleId\":21,\"M_AlarmCode\":331, \"M_Command\":4,\"M_EnergyChannelId\":0,\"M_Message\":\"HELP\", \"M_CommandParams\":\"\",\"M_CommandOptions\":\"\"}", "{\"Partition\":\"CAMM_INTERNAL_EXT_P4_Unit_20\",\"M_AudioSequence\":1,\"Message\":\"DftAudioPlayCommand\",\"M_PlayMode\":3,\"M_Priority\":0,\"M_Volume\":50,\"M_OverrideSeqVolume\":false}", "{\"M_EnergyChannelId\":3,\"Partition\":\"CAMM_INTERNAL_EXT_P4_Unit_20\",\"Message\":\"DftInstrumentCommand\",\"M_DftInstrumentCommand\":1,\"M_IntValue\":0,\"M_FloatValue\":0.0,\"M_StringValue\":\"\"}", "{\"Partition\":\"CAMM_EXT_1078620_AC143800015\",\"Message\":\"DftLogCommand\",\"M_Command\":3,\"M_CommandOptions\":\"\"}", "{\"M_Command\":1,\"M_CalibrationType\":0,\"M_CalibrationTime\":\"\",\"M_Options\":\"\",\"M_EmA2dCalData.M_BipLowCurrentSecondary.M_Offset\":0.0,\"M_EmA2dCalData.M_BipLowCurrentPrimary.M_Gain\":1.0, \"M_EmA2dCalData.M_BipLowVoltPrimary.M_Gain\":1.0,\"Partition\":\"CAMM_INTERNAL_EXT_P4_Unit_20\",\"M_EmA2dCalData.M_BipHighVoltSecondary.M_Offset\":0.0,\"M_EmA2dCalData.M_BipLowVoltSecondary.M_Gain\":1.0, \"M_EmA2dCalData.M_BipLowVoltPrimary.M_Offset\":0.0,\"M_EmA2dCalData.M_BipHighVoltPrimary.M_Gain\":1.0,\"M_EmA2dCalData.M_MonoLowVoltPrimary.M_Offset\":0.0, \"M_EmA2dCalData.M_MonoLowVoltSecondary.M_Offset\":0.0,\"M_EmA2dCalData.M_BipHighCurrentSecondary.M_Offset\":0.0,\"M_EmA2dCalData.M_MonoLowVoltSecondary.M_Gain\":1.0, \"M_EmA2dCalData.M_BipHighCurrentPrimary.M_Gain\":1.0,\"M_EmA2dCalData.M_BipHighVoltSecondary.M_Gain\":1.0,\"M_EmA2dCalData.M_MonoHighVoltSecondary.M_Offset\":0.0, \"M_EmA2dCalData.M_BipHighCurrentPrimary.M_Offset\":0.0,\"Message\":\"EmA2dCalDataCommand\",\"M_EmA2dCalData.M_BipLowCurrentSecondary.M_Gain\":1.0, \"M_EmA2dCalData.M_BipLowCurrentPrimary.M_Offset\":0.0,\"M_EmA2dCalData.M_MonoHighVoltPrimary.M_Gain\":1.0, \"M_EmA2dCalData.M_BipHighCurrentSecondary.M_Gain\":1.0,\"M_EmA2dCalData.M_MonoHighVoltSecondary.M_Gain\":1.0, \"M_EmA2dCalData.M_BipHighVoltPrimary.M_Offset\":0.0,\"M_EmA2dCalData.M_MonoLowVoltPrimary.M_Gain\":1.0, \"M_EmA2dCalData.M_MonoHighVoltPrimary.M_Offset\":0.0,\"M_EmA2dCalData.M_BipLowVoltSecondary.M_Offset\":0.0}", "{\"M_EmA2dCalData.M_BipLowCurrentSecondary.M_Offset\":0.0,\"M_EmA2dCalData.M_BipLowCurrentPrimary.M_Gain\":1.01491,\"M_EmA2dCalData.M_BipLowVoltPrimary.M_Gain\":1.03926, \"Partition\":\"CAMM_EXT_1078620_AC143800029\",\"M_EmA2dCalData.M_BipHighVoltSecondary.M_Offset\":0.0,\"M_EmA2dCalData.M_BipLowVoltPrimary.M_Offset\":0.0, \"M_EmA2dCalData.M_BipLowVoltSecondary.M_Gain\":1.02606,\"M_EmA2dCalData.M_BipHighVoltPrimary.M_Gain\":1.03662,\"M_EmA2dCalData.M_MonoLowVoltPrimary.M_Offset\":0.0, \"M_EmA2dCalData.M_MonoLowVoltSecondary.M_Offset\":0.0,\"M_EmA2dCalData.M_BipHighCurrentSecondary.M_Offset\":0.0,\"M_EmA2dCalData.M_MonoLowVoltSecondary.M_Gain\":1.05138, \"M_EmA2dCalData.M_BipHighCurrentPrimary.M_Gain\":1.01475,\"M_EmA2dCalData.M_BipHighVoltSecondary.M_Gain\":1.02351,\"M_EmA2dCalData.M_MonoHighVoltSecondary.M_Offset\":0.0, \"M_EmA2dCalData.M_BipHighCurrentPrimary.M_Offset\":0.0,\"Message\":\"EmA2dCalDataStatus\",\"M_EmA2dCalData.M_BipLowCurrentSecondary.M_Gain\":1.0347, \"M_EmA2dCalData.M_BipLowCurrentPrimary.M_Offset\":0.0,\"M_EmA2dCalData.M_MonoHighVoltPrimary.M_Gain\":1.07264,\"M_EmA2dCalData.M_MonoHighVoltSecondary.M_Gain\":1.05568, \"M_EmA2dCalData.M_BipHighCurrentSecondary.M_Gain\":1.03478,\"M_Options\":\"\",\"M_EmA2dCalData.M_BipHighVoltPrimary.M_Offset\":0.0, \"M_CalibrationTime\":\"2014-11-18T00:26:27Z\", \"M_EmA2dCalData.M_MonoLowVoltPrimary.M_Gain\":1.06396,\"M_EmA2dCalData.M_MonoHighVoltPrimary.M_Offset\":0.0, \"M_CalibrationType\":-1,\"M_EmA2dCalData.M_BipLowVoltSecondary.M_Offset\":0.0}", "{\"Message\":\"EnergyParameterCommand\",\"Partition\":\"CAMM_EXT_1078620_AC143800015\",\"M_EnergyChannelId\":0;,\"M_InstrumentType\":1;,\"M_ParameterType\":1,\"M_ParameterValue\":3,\"M_EnergyMode\":-1}", "{\"Message\":\"ExternalCommCommand\",\"Partition\":\"CAMM_EXT_1078620_AC143800015\",\"M_ControllerBoardId\":\"1078620_AC143800015\",\"M_ClientId\":\"\",\"M_Command\":5,\"M_CommandOptions\":\"\"}"] ("String") -> [w291]
    stop <- w293 stop-if-true
    n140 = Dequeue Element(queue=w298) -> (element=w299:T41)  [unwired: 2 in, 3 out]
    n141 = Unbundle By Name(w299) -> ("Message"=w297:string, "Message Data"=w296:variant)
    n142 = case shown="\"Bipolar Mode\"" w297 {
      tunnel: w296 -> [_ _ _ _ _ _ _ _ _ _ w404 w569 _ _ w598 w609 _ _ w639 w649 _ _ w679 w689 _ _ w719 w729 _ _ w759 w769 _]
      tunnel: [w306 w310 w323 w332 w344 w355 w365 w376 w388 w397 w407 w566 w573 w591 w600 w605 w619 w631 w640 w644 w659 w671 w680 w683 w699 w711 w720 w723 w739 w751 w760 w764 w771] -> w295
      tunnel: w294 -> [w306 w311 w324 w333 w345 w356 w366 w377 w389 w398 w408 w567 w574 w592 w601 w606 w620 w632 w641 w645 w660 w672 w681 w684 w700 w712 w721 w725 w740 w752 w761 w766 w771]
      tunnel: [FALSE FALSE FALSE FALSE FALSE FALSE FALSE FALSE FALSE FALSE FALSE FALSE FALSE FALSE FALSE FALSE FALSE FALSE FALSE FALSE FALSE FALSE FALSE FALSE FALSE FALSE FALSE FALSE FALSE FALSE FALSE FALSE TRUE] -> w293
      tunnel: [w304 w307 w319 w329 w334 w353 w363 w374 w386 w395 w406 w565 w571 w583 w595 w608 w618 w630 w638 w648 w658 w670 w678 w688 w698 w710 w718 w728 w738 w750 w758 w768 w770] -> w292
      tunnel: w291 -> [w304 w307 w319 w329 w334 w353 w363 w374 w386 w395 w406 w565 w571 w583 w595 w608 w618 w630 w638 w648 w658 w670 w678 w688 w698 w710 w718 w728 w738 w750 w758 w768 w770]
      frame "Init", Default {
        w303 = "Initialization Complete. Ready for Commands" ("Display Message")
        n143 = property on="Port" class="Enum (strict)"("Val(Sgnl)"=enum16{"Mono1", "Mono2", "Bipolar", "Ligasure"}."Mono1" ("Value (Signaling)")) -> (error out=w300:errorcluster)  [unwired: 2 in, 1 out]
        n144 = local write "Display Message page 2"(w303) -> ()
        n145 = local write "Display Message"(w303) -> ()
        n146 = property on="Mode" class="Enum (strict)"(error in=w300, "Val(Sgnl)"=enum16{"Cut", "Coag", "Bipolar", "Ligasure"}."Cut" ("Value (Signaling)")) -> ()  [unwired: 1 in, 2 out]
      }
      frame "Fornax Action 1" {
        n147 = call "FT10_Fornax Command.vi"("ExternalCommCommand"="ExternalCommCommand") -> ("JSON Message"=w313:string)  [unwired: 10 in]
        n148 = local write "Display Message"("\"Action 1\" button pressed" ("Display Message")) -> ()
        n149 = TCP Write(connection ID=w311, data in=w313, 9:100 ("timeout ms (25000)")) -> (connection ID out=w310:refnum<k5>)  [unwired: 1 in, 2 out]
      }
      frame "Send String Array Command" {
        n150 = Index Array(array=w319, index="Numeric (0-8)") -> (element=w315:string)
        "String" <- w315
        n151 = TCP Write(connection ID=w324, data in=w315, 9:100 ("timeout ms (25000)")) -> (connection ID out=w323:refnum<k5>, error out=w317:errorcluster)  [unwired: 1 in, 1 out]
        n152 = local write "Display Message page 2"(w315) -> ()
        n153 = Unbundle By Name(w317) -> ("status"=→"status":bool)
        n154 = local write "Display Message"("\"Send String Array Command\" button pressed" ("Display Message")) -> ()
      }
      frame "Send String Command" {
        n155 = TCP Write(connection ID=w333, data in="String Command", 9:100 ("timeout ms (25000)")) -> (connection ID out=w332:refnum<k5>, error out=w327:errorcluster)  [unwired: 1 in, 1 out]
        n156 = local write "Display Message page 2"("String Command") -> ()
        n157 = Unbundle By Name(w327) -> ("status"=→"status 2":bool)
        n158 = local write "Display Message"("\"Send String Command\" button pressed" ("Display Message")) -> ()
      }
      frame "Fornax Set Monopolar Command" {
        n159 = call "FT10_Fornax MonopolarCommand.vi"("EnergyChannelID"="EnergyChannelID", "Serial Number"="Serial Number", "CutMode"="CutMode", "CoagMode"="CoagMode", "CutPowerCommand"="CutPowerCommand", "CoagPowerCommand"="CoagPowerCommand") -> ("JSON Command"=w341:string)  [unwired: 9 in]
        n160 = local write "Display Message"("\"Set Monopolar Command\" button pressed" ("Display Message")) -> ()
        n161 = TCP Write(connection ID=w345, data in=w341, 9:100 ("timeout ms (25000)")) -> (connection ID out=w344:refnum<k5>)  [unwired: 1 in, 2 out]
      }
      frame "External Command" {
        n162 = Number To Decimal String(number="External Command") -> (decimal integer string=w351:string)  [unwired: 1 in]
        n163 = Concatenate Strings("{\"Message\":\"ExternalCommCommand\",\"Partition\":\"CAMM_EXT_1234321_AJ142800009\",\"M_ControllerBoardId\":\"1234321_AJ142800009\",\"M_ClientId\":\"\",\"M_Command\":", w351, ",\"M_CommandOptions\":\"\"}") -> (w348:string)
        n164 = TCP Write(connection ID=w356, data in=w348, 9:100 ("timeout ms (25000)")) -> (connection ID out=w355:refnum<k5>)  [unwired: 1 in, 2 out]
      }
      frame "System Config" {
        n165 = Number To Decimal String(number="System Config") -> (decimal integer string=w361:string)  [unwired: 1 in]
        n166 = Concatenate Strings("{\"Message\":\"SystemConfigurationCommand\",\"Partition\":\"CAMM_EXT_1234321_AJ142800009\",\"M_ControllerBoardId\":\"1234321_AJ142800009\",\"M_ClientId\":\"\",\"M_Command\":", w361, ",\"M_ConfigurationData\":\"\"}") -> (w358:string)
        n167 = TCP Write(connection ID=w366, data in=w358, 9:100 ("timeout ms (25000)")) -> (connection ID out=w365:refnum<k5>)  [unwired: 1 in, 2 out]
      }
      frame "Switch Status Command" {
        n168 = call "FT10_Fornax Switch Status Command.vi"("Generator"=T43 "CAMM_EXT_1234321_AJ142800009", "Switch State"="Switch State", "Energy Channel ID"="Energy Channel ID", "Switch ID"="Switch ID", "Source ID"="Source ID") -> ("JSON Command"=w367:string)  [unwired: 6 in]
        n169 = TCP Write(connection ID=w377, data in=w367, 9:100 ("timeout ms (25000)")) -> (connection ID out=w376:refnum<k5>)  [unwired: 1 in, 2 out]
      }
      frame "Energy Parameter Command" {
        n170 = call "FT10_Fornax Energy Parameter Command.vi"("Energy Channel ID"="Energy Channel ID 3", "Generator"=T43 "CAMM_EXT_1234321_AJ1428000", "Instrument Type"="Instrument Type", "Parameter Type"="Parameter Type", "Parameter Value"="Parameter Value", "Energy Mode"="Energy Mode") -> ("JSON Command"=w378:string)  [unwired: 9 in]
        n171 = TCP Write(connection ID=w389, data in=w378, 9:100 ("timeout ms (25000)")) -> (connection ID out=w388:refnum<k5>)  [unwired: 1 in, 2 out]
      }
      frame "Slider Status Command" {
        n172 = call "FT10_Fornax Slider Status Command.vi"("Slider Position"="Slider Position", "Energy Channel ID"="Energy Channel ID 2", "Generator"=T43 "CAMM_EXT_1234321_AJ142800009") -> ("JSON Command"=w393:string)  [unwired: 8 in]
        n173 = TCP Write(connection ID=w398, data in=w393, 9:100 ("timeout ms (25000)")) -> (connection ID out=w397:refnum<k5>)  [unwired: 1 in, 2 out]
      }
      frame "Activate Port" {
        n174 = Variant To Data(type=T42 {"Port"=enum."Bipolar", "Mode"=enum."Bipolar", "On/Off"=FALSE}, Variant=w404) -> (data=w402:T42)  [unwired: 1 in, 1 out]
        n175 = Unbundle By Name(w402) -> ("Port"=w401:enum16{"Mono1", "Mono2", "Bipolar", "Ligasure"}, "Mode"=w400:enum16{"Cut", "Coag", "Bipolar", "Ligasure"}, "On/Off"=w399:bool)
        n176 = case shown="\"Mono2\"" w401 {
          selector: w401 -> [w411 w460 w509 w537]
          tunnel: w408 -> [w413 w462 w511 w539]
          tunnel: [w412 w461 w510 w538] -> w407
          tunnel: w400 -> [w410 w459 w508 w536]
          tunnel: w399 -> [w409 w458 w507 w535]
          frame "Mono2" {
            n177 = case shown="\"Cut\"" w410 {
              tunnel: w413 -> [w416 w437 w457]
              tunnel: [w415 w436 w457] -> w412
              tunnel: w411 -> [_ _ _]
              tunnel: w409 -> [w414 w435 _]
              frame "Coag" {
                n178 = case shown="True" w414 {
                  tunnel: w416 -> [w425 w434]
                  tunnel: [w424 w433] -> w415
                  frame True {
                    n179 = call "FT10_Fornax Switch Status Command.vi"("Generator"=T43 "CAMM_EXT_1234321_AJ142800009", "Switch State"=Control_Fornax_Switch_State."SWITCH_STATE_PRESSED  ", "Energy Channel ID"=Control_Fornax_Energy_Channel_ID."EC_MONO_2  ", "Switch ID"=Control_Fornax_Switch_ID."SWITCH_ID_COAG  ", "Source ID"=Control_Fornax_Source_ID."SWITCH_SOURCE_HANDSWITCH  ") -> ("JSON Command"=w417:string)  [unwired: 6 in]
                    n180 = TCP Write(connection ID=w425, data in=w417, 9:100 ("timeout ms (25000)")) -> (connection ID out=w424:refnum<k5>)  [unwired: 1 in, 2 out]
                  }
                  frame False {
                    n181 = call "FT10_Fornax Switch Status Command.vi"("Generator"=T43 "CAMM_EXT_1234321_AJ142800009", "Switch State"=Control_Fornax_Switch_State."SWITCH_STATE_RELEASED  ", "Energy Channel ID"=Control_Fornax_Energy_Channel_ID."EC_MONO_2  ", "Switch ID"=Control_Fornax_Switch_ID."SWITCH_ID_COAG  ", "Source ID"=Control_Fornax_Source_ID."SWITCH_SOURCE_HANDSWITCH  ") -> ("JSON Command"=w426:string)  [unwired: 6 in]
                    n182 = TCP Write(connection ID=w434, data in=w426, 9:100 ("timeout ms (25000)")) -> (connection ID out=w433:refnum<k5>)  [unwired: 1 in, 2 out]
                  }
                }
              }
              frame "Cut" {
                n183 = case shown="True" w435 {
                  tunnel: w437 -> [w446 w455]
                  tunnel: [w445 w454] -> w436
                  frame True {
                    n184 = call "FT10_Fornax Switch Status Command.vi"("Generator"=T43 "CAMM_EXT_1234321_AJ142800009", "Switch State"=Control_Fornax_Switch_State."SWITCH_STATE_PRESSED  ", "Energy Channel ID"=Control_Fornax_Energy_Channel_ID."EC_MONO_2  ", "Switch ID"=Control_Fornax_Switch_ID."SWITCH_ID_CUT  ", "Source ID"=Control_Fornax_Source_ID."SWITCH_SOURCE_HANDSWITCH  ") -> ("JSON Command"=w438:string)  [unwired: 6 in]
                    n185 = TCP Write(connection ID=w446, data in=w438, 9:100 ("timeout ms (25000)")) -> (connection ID out=w445:refnum<k5>)  [unwired: 1 in, 2 out]
                  }
                  frame False {
                    n186 = call "FT10_Fornax Switch Status Command.vi"("Generator"=T43 "CAMM_EXT_1234321_AJ142800009", "Switch State"=Control_Fornax_Switch_State."SWITCH_STATE_RELEASED  ", "Energy Channel ID"=Control_Fornax_Energy_Channel_ID."EC_MONO_2  ", "Switch ID"=Control_Fornax_Switch_ID."SWITCH_ID_CUT  ", "Source ID"=Control_Fornax_Source_ID."SWITCH_SOURCE_HANDSWITCH  ") -> ("JSON Command"=w447:string)  [unwired: 6 in]
                    n187 = TCP Write(connection ID=w455, data in=w447, 9:100 ("timeout ms (25000)")) -> (connection ID out=w454:refnum<k5>)  [unwired: 1 in, 2 out]
                  }
                }
              }
              frame Default {
                n188 = One Button Dialog(message="This mode is not allowed for this port") -> ()  [unwired: 1 in, 1 out]
              }
            }
          }
          frame "Mono1" {
            n189 = case shown="\"Coag\"" w459 {
              tunnel: w462 -> [w465 w486 w506]
              tunnel: [w464 w485 w506] -> w461
              tunnel: w460 -> [_ _ _]
              tunnel: w458 -> [w463 w484 _]
              frame "Coag" {
                n190 = case shown="False" w463 {
                  tunnel: w465 -> [w474 w483]
                  tunnel: [w473 w482] -> w464
                  frame True {
                    n191 = call "FT10_Fornax Switch Status Command.vi"("Generator"=T43 "CAMM_EXT_1234321_AJ142800009", "Switch State"=Control_Fornax_Switch_State."SWITCH_STATE_PRESSED  ", "Energy Channel ID"=Control_Fornax_Energy_Channel_ID."EC_MONO_1  ", "Switch ID"=Control_Fornax_Switch_ID."SWITCH_ID_COAG  ", "Source ID"=Control_Fornax_Source_ID."SWITCH_SOURCE_HANDSWITCH  ") -> ("JSON Command"=w466:string)  [unwired: 6 in]
                    n192 = TCP Write(connection ID=w474, data in=w466, 9:100 ("timeout ms (25000)")) -> (connection ID out=w473:refnum<k5>)  [unwired: 1 in, 2 out]
                  }
                  frame False {
                    n193 = call "FT10_Fornax Switch Status Command.vi"("Generator"=T43 "CAMM_EXT_1234321_AJ142800009", "Switch State"=Control_Fornax_Switch_State."SWITCH_STATE_RELEASED  ", "Energy Channel ID"=Control_Fornax_Energy_Channel_ID."EC_MONO_1  ", "Switch ID"=Control_Fornax_Switch_ID."SWITCH_ID_COAG  ", "Source ID"=Control_Fornax_Source_ID."SWITCH_SOURCE_HANDSWITCH  ") -> ("JSON Command"=w475:string)  [unwired: 6 in]
                    n194 = TCP Write(connection ID=w483, data in=w475, 9:100 ("timeout ms (25000)")) -> (connection ID out=w482:refnum<k5>)  [unwired: 1 in, 2 out]
                  }
                }
              }
              frame "Cut" {
                n195 = case shown="True" w484 {
                  tunnel: w486 -> [w495 w504]
                  tunnel: [w494 w503] -> w485
                  frame True {
                    n196 = call "FT10_Fornax Switch Status Command.vi"("Generator"=T43 "CAMM_EXT_1234321_AJ142800009", "Switch State"=Control_Fornax_Switch_State."SWITCH_STATE_PRESSED  ", "Energy Channel ID"=Control_Fornax_Energy_Channel_ID."EC_MONO_1  ", "Switch ID"=Control_Fornax_Switch_ID."SWITCH_ID_CUT  ", "Source ID"=Control_Fornax_Source_ID."SWITCH_SOURCE_HANDSWITCH  ") -> ("JSON Command"=w487:string)  [unwired: 6 in]
                    n197 = TCP Write(connection ID=w495, data in=w487, 9:100 ("timeout ms (25000)")) -> (connection ID out=w494:refnum<k5>)  [unwired: 1 in, 2 out]
                  }
                  frame False {
                    n198 = call "FT10_Fornax Switch Status Command.vi"("Generator"=T43 "CAMM_EXT_1234321_AJ142800009", "Switch State"=Control_Fornax_Switch_State."SWITCH_STATE_RELEASED  ", "Energy Channel ID"=Control_Fornax_Energy_Channel_ID."EC_MONO_1  ", "Switch ID"=Control_Fornax_Switch_ID."SWITCH_ID_CUT  ", "Source ID"=Control_Fornax_Source_ID."SWITCH_SOURCE_HANDSWITCH  ") -> ("JSON Command"=w496:string)  [unwired: 6 in]
                    n199 = TCP Write(connection ID=w504, data in=w496, 9:100 ("timeout ms (25000)")) -> (connection ID out=w503:refnum<k5>)  [unwired: 1 in, 2 out]
                  }
                }
              }
              frame Default {
                n200 = One Button Dialog(message="This mode is not allowed for this port") -> ()  [unwired: 1 in, 1 out]
              }
            }
          }
          frame "Bipolar" {
            n201 = case shown="\"Bipolar\"" w508 {
              tunnel: w511 -> [w514 w534]
              tunnel: [w513 w534] -> w510
              tunnel: w509 -> [_ _]
              tunnel: w507 -> [w512 _]
              frame "Bipolar" {
                n202 = case shown="False" w512 {
                  tunnel: w514 -> [w523 w532]
                  tunnel: [w522 w531] -> w513
                  frame True {
                    n203 = call "FT10_Fornax Switch Status Command.vi"("Generator"=T43 "CAMM_EXT_1234321_AJ142800009", "Switch State"=Control_Fornax_Switch_State."SWITCH_STATE_PRESSED  ", "Energy Channel ID"=Control_Fornax_Energy_Channel_ID."EC_BIPOLAR  ", "Switch ID"=Control_Fornax_Switch_ID."SWITCH_ID_BIPOLAR  ", "Source ID"=Control_Fornax_Source_ID."SWITCH_SOURCE_HANDSWITCH  ") -> ("JSON Command"=w515:string)  [unwired: 6 in]
                    n204 = TCP Write(connection ID=w523, data in=w515, 9:100 ("timeout ms (25000)")) -> (connection ID out=w522:refnum<k5>)  [unwired: 1 in, 2 out]
                  }
                  frame False {
                    n205 = call "FT10_Fornax Switch Status Command.vi"("Generator"=T43 "CAMM_EXT_1234321_AJ142800009", "Switch State"=Control_Fornax_Switch_State."SWITCH_STATE_RELEASED  ", "Energy Channel ID"=Control_Fornax_Energy_Channel_ID."EC_BIPOLAR  ", "Switch ID"=Control_Fornax_Switch_ID."SWITCH_ID_BIPOLAR  ", "Source ID"=Control_Fornax_Source_ID."SWITCH_SOURCE_HANDSWITCH  ") -> ("JSON Command"=w524:string)  [unwired: 6 in]
                    n206 = TCP Write(connection ID=w532, data in=w524, 9:100 ("timeout ms (25000)")) -> (connection ID out=w531:refnum<k5>)  [unwired: 1 in, 2 out]
                  }
                }
              }
              frame Default {
                n207 = One Button Dialog(message="This mode is not allowed for this port") -> ()  [unwired: 1 in, 1 out]
              }
            }
          }
          frame "Ligasure" {
            n208 = case shown="\"Ligasure\"" w536 {
              tunnel: w539 -> [w542 w562]
              tunnel: [w541 w562] -> w538
              tunnel: w537 -> [_ _]
              tunnel: w535 -> [w540 _]
              frame "Ligasure" {
                n209 = case shown="True" w540 {
                  tunnel: w542 -> [w551 w560]
                  tunnel: [w550 w559] -> w541
                  frame True {
                    n210 = call "FT10_Fornax Switch Status Command.vi"("Generator"=T43 "CAMM_EXT_1234321_AJ142800009", "Switch State"=Control_Fornax_Switch_State."SWITCH_STATE_PRESSED  ", "Energy Channel ID"=Control_Fornax_Energy_Channel_ID."EC_ADVANCED  ", "Switch ID"=Control_Fornax_Switch_ID."SWITCH_ID_LIGASURE  ", "Source ID"=Control_Fornax_Source_ID."SWITCH_SOURCE_HANDSWITCH  ") -> ("JSON Command"=w543:string)  [unwired: 6 in]
                    n211 = TCP Write(connection ID=w551, data in=w543, 9:100 ("timeout ms (25000)")) -> (connection ID out=w550:refnum<k5>)  [unwired: 1 in, 2 out]
                  }
                  frame False {
                    n212 = call "FT10_Fornax Switch Status Command.vi"("Generator"=T43 "CAMM_EXT_1234321_AJ142800009", "Switch State"=Control_Fornax_Switch_State."SWITCH_STATE_RELEASED  ", "Energy Channel ID"=Control_Fornax_Energy_Channel_ID."EC_ADVANCED  ", "Switch ID"=Control_Fornax_Switch_ID."SWITCH_ID_LIGASURE  ", "Source ID"=Control_Fornax_Source_ID."SWITCH_SOURCE_HANDSWITCH  ") -> ("JSON Command"=w552:string)  [unwired: 6 in]
                    n213 = TCP Write(connection ID=w560, data in=w552, 9:100 ("timeout ms (25000)")) -> (connection ID out=w559:refnum<k5>)  [unwired: 1 in, 2 out]
                  }
                }
              }
              frame Default {
                n214 = One Button Dialog(message="This mode is not allowed for this port") -> ()  [unwired: 1 in, 1 out]
              }
            }
          }
        }
      }
      frame "Bipolar Activate Port" {
        n215 = Variant To Data(type=T21 FALSE ("Bipolar Activate"), Variant=w569) -> (data=w568:T21)  [unwired: 1 in, 1 out]
        n216 = call "FT10_Fornax Bipolar Activate Port Command.vi"("Bipolar Activate"=w568, "TCP Network Connection in"=w567) -> ("TCP Network Connection out"=w566:refnum<k5>)  [unwired: 9 in]
      }
      frame "Bipolar Decrease Power" {
        # "Decrease Bipolar Power"
        n217 = call "FT10_Fornax Energy Parameter Command.vi"("Energy Channel ID"=Control_Fornax_Energy_Channel_ID."EC_BIPOLAR  ", "Generator"=T43 "CAMM_EXT_1234321_AJ1428000", "Instrument Type"=Control_Fornax_Instrument_Type."INSTRUMENT_TYPE_BIPOLAR", "Parameter Type"=Control_Fornax_Parameter_Type."POWER_PARAMETER", "Parameter Value"=T19 2, "Energy Mode"=Control_Fornax_Energy_Mode."BIPOLAR_MODE") -> ("JSON Command"=w572:string)  [unwired: 9 in]
        n218 = TCP Write(connection ID=w574, data in=w572, 9:100 ("timeout ms (25000)")) -> (connection ID out=w573:refnum<k5>)  [unwired: 1 in, 2 out]
      }
      frame "Bipolar Increase Power" {
        # "Increase Bipolar Power"
        n219 = call "FT10_Fornax Energy Parameter Command.vi"("Energy Channel ID"=Control_Fornax_Energy_Channel_ID."EC_BIPOLAR  ", "Generator"=T43 "CAMM_EXT_1234321_AJ1428000", "Instrument Type"=Control_Fornax_Instrument_Type."INSTRUMENT_TYPE_BIPOLAR", "Parameter Type"=Control_Fornax_Parameter_Type."POWER_PARAMETER", "Parameter Value"=T19 1, "Energy Mode"=Control_Fornax_Energy_Mode."BIPOLAR_MODE") -> ("JSON Command"=w584:string)  [unwired: 9 in]
        n220 = TCP Write(connection ID=w592, data in=w584, 9:100 ("timeout ms (25000)")) -> (connection ID out=w591:refnum<k5>)  [unwired: 1 in, 2 out]
      }
      frame "Bipolar Mode" {
        n221 = Variant To Data(type=Control_Fornax_Bipolar_Enum."Standard" ("Bipolar Enum"), Variant=w598) -> (data=w596:T22)  [unwired: 1 in, 1 out]
        n222 = call "FT10_Fornax Bipolar Mode Command.vi"("Bipolar Enum"=w596) -> ("JSON Command"=w599:string)  [unwired: 10 in]
        n223 = TCP Write(connection ID=w601, data in=w599, 9:100 ("timeout ms (25000)")) -> (connection ID out=w600:refnum<k5>)  [unwired: 1 in, 2 out]
      }
      frame "Mono1 Cut Activate Port" {
        n224 = Variant To Data(type=T34 FALSE ("Mono1 Cut Activate"), Variant=w609) -> (data=w604:T34)  [unwired: 1 in, 1 out]
        n225 = call "FT10_Fornax Mono1 Cut Activate Port Command.vi"("Mono1 Cut Activate"=w604, "TCP Network Connection in"=w606) -> ("TCP Network Connection out"=w605:refnum<k5>)  [unwired: 9 in]
      }
      frame "Mono1 Cut Decrease Power" {
        # "Decrease Mono1 Cut Power"
        n226 = call "FT10_Fornax Energy Parameter Command.vi"("Energy Channel ID"=Control_Fornax_Energy_Channel_ID."EC_MONO_1  ", "Generator"=T43 "CAMM_EXT_1234321_AJ1428000", "Instrument Type"=Control_Fornax_Instrument_Type."INSTRUMENT_TYPE_MONOPOLAR", "Parameter Type"=Control_Fornax_Parameter_Type."CUT_MODALITY_POWER_PARAMETER", "Parameter Value"=T19 2, "Energy Mode"=Control_Fornax_Energy_Mode."CUT_MODE") -> ("JSON Command"=w610:string)  [unwired: 9 in]
        n227 = TCP Write(connection ID=w620, data in=w610, 9:100 ("timeout ms (25000)")) -> (connection ID out=w619:refnum<k5>)  [unwired: 1 in, 2 out]
      }
      frame "Mono1 Cut Increase Power" {
        # "Increase Mono1 Cut Power"
        n228 = call "FT10_Fornax Energy Parameter Command.vi"("Energy Channel ID"=Control_Fornax_Energy_Channel_ID."EC_MONO_1  ", "Generator"=T43 "CAMM_EXT_1234321_AJ1428000", "Instrument Type"=Control_Fornax_Instrument_Type."INSTRUMENT_TYPE_MONOPOLAR", "Parameter Type"=Control_Fornax_Parameter_Type."CUT_MODALITY_POWER_PARAMETER", "Parameter Value"=T19 1, "Energy Mode"=Control_Fornax_Energy_Mode."CUT_MODE") -> ("JSON Command"=w622:string)  [unwired: 9 in]
        n229 = TCP Write(connection ID=w632, data in=w622, 9:100 ("timeout ms (25000)")) -> (connection ID out=w631:refnum<k5>)  [unwired: 1 in, 2 out]
      }
      frame "Mono1 Cut Mode" {
        n230 = Variant To Data(type=Control_Fornax_Mono1_Cut_Enum."Pure" ("Mono1 Cut Enum"), Variant=w639) -> (data=w636:T36)  [unwired: 1 in, 1 out]
        n231 = call "FT10_Fornax Mono1 Cut Mode Command.vi"("Mono1 Cut Enum"=w636) -> ("JSON Command"=w635:string)  [unwired: 10 in]
        n232 = TCP Write(connection ID=w641, data in=w635, 9:100 ("timeout ms (25000)")) -> (connection ID out=w640:refnum<k5>)  [unwired: 1 in, 2 out]
      }
      frame "Mono1 Coag Activate Port" {
        n233 = Variant To Data(type=T33 FALSE ("Mono1 Coag Activate"), Variant=w649) -> (data=w643:T33)  [unwired: 1 in, 1 out]
        n234 = call "FT10_Fornax Mono1 Coag Activate Port Command.vi"("Mono1 Coag Activate"=w643, "TCP Network Connection in"=w645) -> ("TCP Network Connection out"=w644:refnum<k5>)  [unwired: 9 in]
      }
      frame "Mono1 Coag Decrease Power" {
        # "Decrease Mono1 Coag Power"
        n235 = call "FT10_Fornax Energy Parameter Command.vi"("Energy Channel ID"=Control_Fornax_Energy_Channel_ID."EC_MONO_1  ", "Generator"=T43 "CAMM_EXT_1234321_AJ1428000", "Instrument Type"=Control_Fornax_Instrument_Type."INSTRUMENT_TYPE_MONOPOLAR", "Parameter Type"=Control_Fornax_Parameter_Type."COAG_MODALITY_POWER_PARAMETER", "Parameter Value"=T19 2, "Energy Mode"=Control_Fornax_Energy_Mode."FULGERATE_MODE") -> ("JSON Command"=w650:string)  [unwired: 9 in]
        n236 = TCP Write(connection ID=w660, data in=w650, 9:100 ("timeout ms (25000)")) -> (connection ID out=w659:refnum<k5>)  [unwired: 1 in, 2 out]
      }
      frame "Mono1 Coag Increase Power" {
        # "Increase Mono1 Coag Power"
        n237 = call "FT10_Fornax Energy Parameter Command.vi"("Energy Channel ID"=Control_Fornax_Energy_Channel_ID."EC_MONO_1  ", "Generator"=T43 "CAMM_EXT_1234321_AJ1428000", "Instrument Type"=Control_Fornax_Instrument_Type."INSTRUMENT_TYPE_MONOPOLAR", "Parameter Type"=Control_Fornax_Parameter_Type."COAG_MODALITY_POWER_PARAMETER", "Parameter Value"=T19 1, "Energy Mode"=Control_Fornax_Energy_Mode."FULGERATE_MODE") -> ("JSON Command"=w662:string)  [unwired: 9 in]
        n238 = TCP Write(connection ID=w672, data in=w662, 9:100 ("timeout ms (25000)")) -> (connection ID out=w671:refnum<k5>)  [unwired: 1 in, 2 out]
      }
      frame "Mono1 Coag Mode" {
        n239 = Variant To Data(type=Control_Fornax_Mono1_Coag_Enum."Fulgerate" ("Mono1 Coag Enum"), Variant=w679) -> (data=w676:T35)  [unwired: 1 in, 1 out]
        n240 = call "FT10_Fornax Mono1 Coag Mode Command.vi"("Mono1 Coag Enum"=w676) -> ("JSON Command"=w675:string)  [unwired: 10 in]
        n241 = TCP Write(connection ID=w681, data in=w675, 9:100 ("timeout ms (25000)")) -> (connection ID out=w680:refnum<k5>)  [unwired: 1 in, 2 out]
      }
      frame "Mono2 Cut Activate Port" {
        n242 = Variant To Data(type=T32 FALSE ("Mono2 Cut Activate"), Variant=w689) -> (data=w685:T32)  [unwired: 1 in, 1 out]
        n243 = call "FT10_Fornax Mono2 Cut Activate Port Command.vi"("Mono2 Cut Activate"=w685, "TCP Network Connection in"=w684) -> ("TCP Network Connection out"=w683:refnum<k5>)  [unwired: 9 in]
      }
      frame "Mono2 Cut Decrease Power" {
        # "Decrease Mono2 Cut Power"
        n244 = call "FT10_Fornax Energy Parameter Command.vi"("Energy Channel ID"=Control_Fornax_Energy_Channel_ID."EC_MONO_2  ", "Generator"=T43 "CAMM_EXT_1234321_AJ1428000", "Instrument Type"=Control_Fornax_Instrument_Type."INSTRUMENT_TYPE_MONOPOLAR", "Parameter Type"=Control_Fornax_Parameter_Type."CUT_MODALITY_POWER_PARAMETER", "Parameter Value"=T19 2, "Energy Mode"=Control_Fornax_Energy_Mode."CUT_MODE") -> ("JSON Command"=w690:string)  [unwired: 9 in]
        n245 = TCP Write(connection ID=w700, data in=w690, 9:100 ("timeout ms (25000)")) -> (connection ID out=w699:refnum<k5>)  [unwired: 1 in, 2 out]
      }
      frame "Mono2 Cut Increase Power" {
        # "Increase Mono2 Cut Power"
        n246 = call "FT10_Fornax Energy Parameter Command.vi"("Energy Channel ID"=Control_Fornax_Energy_Channel_ID."EC_MONO_2  ", "Generator"=T43 "CAMM_EXT_1234321_AJ1428000", "Instrument Type"=Control_Fornax_Instrument_Type."INSTRUMENT_TYPE_MONOPOLAR", "Parameter Type"=Control_Fornax_Parameter_Type."CUT_MODALITY_POWER_PARAMETER", "Parameter Value"=T19 1, "Energy Mode"=Control_Fornax_Energy_Mode."CUT_MODE") -> ("JSON Command"=w702:string)  [unwired: 9 in]
        n247 = TCP Write(connection ID=w712, data in=w702, 9:100 ("timeout ms (25000)")) -> (connection ID out=w711:refnum<k5>)  [unwired: 1 in, 2 out]
      }
      frame "Mono2 Cut Mode" {
        n248 = Variant To Data(type=Control_Fornax_Mono2_Cut_Enum."Pure" ("Mono2 Cut Enum"), Variant=w719) -> (data=w715:T28)  [unwired: 1 in, 1 out]
        n249 = call "FT10_Fornax Mono2 Cut Mode Command.vi"("Mono2 Cut Enum"=w715) -> ("JSON Command"=w714:string)  [unwired: 10 in]
        n250 = TCP Write(connection ID=w721, data in=w714, 9:100 ("timeout ms (25000)")) -> (connection ID out=w720:refnum<k5>)  [unwired: 1 in, 2 out]
      }
      frame "Mono2 Coag Activate Port" {
        n251 = Variant To Data(type=T31 FALSE ("Mono2 Coag Activate"), Variant=w729) -> (data=w724:T31)  [unwired: 1 in, 1 out]
        n252 = call "FT10_Fornax Mono2 Coag Activate Port Command.vi"("Mono2 Coag Activate"=w724, "TCP Network Connection in"=w725) -> ("TCP Network Connection out"=w723:refnum<k5>)  [unwired: 9 in]
      }
      frame "Mono2 Coag Decrease Power" {
        # "Decrease Mono2 Coag Power"
        n253 = call "FT10_Fornax Energy Parameter Command.vi"("Energy Channel ID"=Control_Fornax_Energy_Channel_ID."EC_MONO_2  ", "Generator"=T43 "CAMM_EXT_1234321_AJ1428000", "Instrument Type"=Control_Fornax_Instrument_Type."INSTRUMENT_TYPE_MONOPOLAR", "Parameter Type"=Control_Fornax_Parameter_Type."COAG_MODALITY_POWER_PARAMETER", "Parameter Value"=T19 2, "Energy Mode"=Control_Fornax_Energy_Mode."FULGERATE_MODE") -> ("JSON Command"=w730:string)  [unwired: 9 in]
        n254 = TCP Write(connection ID=w740, data in=w730, 9:100 ("timeout ms (25000)")) -> (connection ID out=w739:refnum<k5>)  [unwired: 1 in, 2 out]
      }
      frame "Mono2 Coag Increase Power" {
        # "Increase Mono2 Coag Power"
        n255 = call "FT10_Fornax Energy Parameter Command.vi"("Energy Channel ID"=Control_Fornax_Energy_Channel_ID."EC_MONO_2  ", "Generator"=T43 "CAMM_EXT_1234321_AJ1428000", "Instrument Type"=Control_Fornax_Instrument_Type."INSTRUMENT_TYPE_MONOPOLAR", "Parameter Type"=Control_Fornax_Parameter_Type."COAG_MODALITY_POWER_PARAMETER", "Parameter Value"=T19 1, "Energy Mode"=Control_Fornax_Energy_Mode."FULGERATE_MODE") -> ("JSON Command"=w742:string)  [unwired: 9 in]
        n256 = TCP Write(connection ID=w752, data in=w742, 9:100 ("timeout ms (25000)")) -> (connection ID out=w751:refnum<k5>)  [unwired: 1 in, 2 out]
      }
      frame "Mono2 Coag Mode" {
        n257 = Variant To Data(type=Control_Fornax_Mono2_Coag_Enum."Fulgerate" ("Mono2 Coag Enum"), Variant=w759) -> (data=w756:T25)  [unwired: 1 in, 1 out]
        n258 = call "FT10_Fornax Mono2 Coag Mode Command.vi"("Mono2 Coag Enum"=w756) -> ("JSON Command"=w755:string)  [unwired: 10 in]
        n259 = TCP Write(connection ID=w761, data in=w755, 9:100 ("timeout ms (25000)")) -> (connection ID out=w760:refnum<k5>)  [unwired: 1 in, 2 out]
      }
      frame "Ligasure Activate Port" {
        n260 = Variant To Data(type=T20 FALSE ("Ligasure Activate"), Variant=w769) -> (data=w765:T20)  [unwired: 1 in, 1 out]
        n261 = call "FT10_Fornax Ligasure Activate Port Command.vi"("Ligasure Activate"=w765, "TCP Network Connection in"=w766) -> ("TCP Network Connection out"=w764:refnum<k5>)  [unwired: 9 in]
      }
      frame "Exit" {
        n262 = local write "Display Message"("\"Stop\" button pressed" ("Display Message")) -> ()
      }
    }
  }
